vi "main_BOC.vi"() -> ()   [LabVIEW 2017]
doc: "Use this template to build a user interface event handler design pattern. Use this pattern for dialog boxes and other user interfaces. You also can create and execute user-defined events that the VI can handle the same way as user interface events."
uses:
  ui.ctl
  classes/dc_power_supply/DC_power_supply.lvclass
  classes/report/Report.lvclass
  ui_buttons.ctl
  types/boc_type.ctl
  types/tolerance_list.ctl
  types/tolerance.ctl
  subVI/motech_power_supply/types/motech_set_value_cluster.ctl
  subVI/motech_power_supply/types/channels_enum.ctl
  Unicorn Labview Library/Control/unicorn_Param.ctl
  Unicorn Labview Library/Control/unicorn_conn.ctl
  Unicorn Labview Library/Control/unicorn_JSON.ctl
  Unicorn Labview Library/Control/unicorn_ParamInt.ctl
  Unicorn Labview Library/Control/unicorn_Telemetry.ctl
  Unicorn Labview Library/Control/unicorn_Table.ctl
  Unicorn Labview Library/Control/unicorn_ParamFloat.ctl
  states_enum.ctl
  classes/dc_power_supply/motech-pps-1200/Motech-pps-1200.lvclass
  types/calibr_table_rows.ctl
  <instrlib>/PICOTEST M352XA/Public/Controls/Function.ctl
  classes/report/Report.lvclass/Report.ctl
  Unicorn Labview Library/Unicorn Library.lvlib
  <instrlib>/Siglent SDG X Series/Siglent SDG X Series.lvlib
panel:
  in  "export_report":bool
  in  "report":path
  in  "template":path
  in  "dc_power_supply":refnum<visa-resource-name>="MOTECH_DC_power_supply" caption="Источник DC"
  in  "channel_timeout_sec":dbl=15.0
  in  "voltmetr":refnum<visa-resource-name>="USB0::0x164E::0x0DAD::TW00054344::INSTR" caption="Вольтметр"
  in  "generator":refnum<visa-resource-name>="generator" caption="Генератор"
  in  "UI":T1
  out "error out":errorcluster
  out "Con":bool
  in  "Tab Control":T4(tab)
  out "Waveform Graph - Dark 2":waveform(sgl)[](graph)
  out "Slide 2":u8(slide) scale=0.0..100.0
  out "Slide":u8(slide) scale=0.0..100.0
  out "Waveform Graph - Dark":waveform(sgl)[](graph)
  in  "VersionControl":bool
  out "output array":sgl[][](array[numeric])
  in  "Array":dbl[][](array[numeric]) format="%_4p"
  in  "calibration":bool
  in  "check_calibr":bool
  in  "tolerance_list":T5=[{"MIN"="-(0.01+0.26*x)", "MAX"="(0.01+0.06*x)"}, {"MIN"="-(0.01+0.09*x)", "MAX"="(0.01+0.06*x)"}, {"MIN"="-(0.01+0.05*x)", "MAX"="(0.01+0.01*x)"}, {"MIN"="-(0.01+0.01*x)", "MAX"="(0.01+0.01*x)"}, {"MIN"="-(0.01+0.01*x)", "MAX"="(0.01+0.01*x)"}, {"MIN"="-(0.01+0.01*x)", "MAX"="(0.01+0.01*x)"}, {"MIN"="-(0.01+0.01*x)", "MAX"="(0.01+0.01*x)"}, {"MIN"="-(0.01+0.11*x)", "MAX"="(0.01+0.01*x)"}]
  in  "freq_values":dbl[](array[numeric])=[0.5, 2.0, 10.0, 20.0, 160.0, 2500.0, 4600.0, 4800.0] caption="Диапозон частот" min=0.0
  in  "freq_character":bool caption="Частотная характеристика"
  out "result_table_freq":dbl[][](array[numeric]) format="%#_4p"
  out "Array 2":bool[][](array[boolean])
  in  "tolerance_list 2":T5=[{"MIN"="-(0.01+0.01*x)", "MAX"="(0.01+0.01*x)"}, {"MIN"="-(0.01+0.01*x)", "MAX"="(0.01+0.01*x)"}, {"MIN"="-(0.01+0.01*x)", "MAX"="(0.01+0.01*x)"}, {"MIN"="-(0.01+0.01*x)", "MAX"="(0.01+0.01*x)"}, {"MIN"="-(0.01+0.01*x)", "MAX"="(0.01+0.01*x)"}, {"MIN"="-(0.01+0.01*x)", "MAX"="(0.01+0.01*x)"}, {"MIN"="-(0.01+0.01*x)", "MAX"="(0.01+0.01*x)"}, {"MIN"="-(0.01+0.01*x)", "MAX"="(0.01+0.01*x)"}]
  in  "volt_values":dbl[](array[numeric])=[5.0, 10.0, 14.0] caption="Диапозон напряжений" min=0.0
  out "check_volt_result":bool[][](array[boolean])
  in  "volt_meas":bool
  out "F-format string 2":string[][](array[string])
  in  "meas_low_voltage_ac_char":bool
  in  "tolerance_list 4":T5=[{"MIN"="-(0.01+0.01*x)", "MAX"="(0.01+0.01*x)"}, {"MIN"="-(0.01+0.01*x)", "MAX"="(0.01+0.01*x)"}, {"MIN"="-(0.01+0.01*x)", "MAX"="(0.01+0.01*x)"}, {"MIN"="-(0.01+0.01*x)", "MAX"="(0.01+0.01*x)"}, {"MIN"="-(0.01+0.01*x)", "MAX"="(0.01+0.01*x)"}, {"MIN"="-(0.01+0.01*x)", "MAX"="(0.01+0.01*x)"}, {"MIN"="-(0.01+0.01*x)", "MAX"="(0.01+0.01*x)"}, {"MIN"="-(0.01+0.01*x)", "MAX"="(0.01+0.01*x)"}]
  in  "volt_values 2":dbl[](array[numeric])=[0.005, 0.1, 1.0] caption="Диапозон напряжений" min=0.0
  out "check_volt_result 2":bool[][](array[boolean])
  out "F-format string":string[][](array[string])
  out "Table Control":string[][](table)
  in  "voltage":dbl[](array[numeric])=[-20.0, -15.0, -10.0, -5.0, -1.0, -0.1, 0.1, 1.0, 5.0, 10.0, 15.0, 20.0]
  in  "dc_voltage_measure":bool caption="connection"
  in  "tolerance_list 3":T5=[{"MIN"="-(0.01+0.01*x)", "MAX"="(0.01+0.01*x)"}, {"MIN"="-(0.01+0.01*x)", "MAX"="(0.01+0.01*x)"}, {"MIN"="-(0.01+0.01*x)", "MAX"="(0.01+0.01*x)"}, {"MIN"="-(0.01+0.01*x)", "MAX"="(0.01+0.01*x)"}, {"MIN"="-(0.01+0.01*x)", "MAX"="(0.01+0.01*x)"}, {"MIN"="-(0.01+0.01*x)", "MAX"="(0.01+0.01*x)"}, {"MIN"="-(0.01+0.01*x)", "MAX"="(0.01+0.01*x)"}, {"MIN"="-(0.01+0.01*x)", "MAX"="(0.01+0.01*x)"}]
  out "Array 3":bool[][](array[boolean])
  in  "set_V":bool
  in  "motech_set_value":T7={"voltage"=0.0, "current"=0.0, "channel"=enum."1"}
  in  "I_control_values":dbl[](array[numeric])=[4.0, 8.0, 12.0, 16.0, 20.0]
  out "first_meas":dbl[](array[numeric])
  out "result_calibration_table":sgl[][](array[numeric])
  out "second_meas":dbl[](array[numeric])
  in  "tolerance_list_I_correction":T5=[{"MIN"="-(0.1+0.01*x*1000)/1000", "MAX"="(0.1+0.01*x*1000)/1000"}, {"MIN"="-(0.1+0.01*x*1000)/1000", "MAX"="(0.1+0.01*x*1000)/1000"}, {"MIN"="-(0.1+0.01*x*1000)/1000", "MAX"="(0.1+0.01*x*1000)/1000"}, {"MIN"="-(0.1+0.01*x*1000)/1000", "MAX"="(0.1+0.01*x*1000)/1000"}, {"MIN"="-(0.1+0.01*x*1000)/1000", "MAX"="(0.1+0.01*x*1000)/1000"}, {"MIN"="-(0.01+0.01*x)", "MAX"="(0.01+0.01*x)"}, {"MIN"="-(0.01+0.01*x)", "MAX"="(0.01+0.01*x)"}, {"MIN"="-(0.01+0.11*x)", "MAX"="(0.01+0.01*x)"}]
  out "check_result":bool[][](array[boolean])
  out "result_table":dbl[][](array[numeric])
  in  "curent_calibr":bool
  in  "avarage_Ac_input":bool
  in  "voltage 2":dbl[](array[numeric])=[20.0, 15.0, 10.0, 5.0, 1.0, 0.1, 0.0, 0.0, 0.0, 0.0, 0.0, 0.0]
  out "Table Control 2":string[][](table)
  in  "check_dc_icp":bool
  out "output array 2":dbl[][](array[numeric]) format="%#_6f"
  out "boc_values":sgl[][](array[numeric]) format="%#_6f"
  in  "connection":bool
  in  "stop":bool
  # "Данные при калибровке"
  # "Проверка калибровки"
  # "dc_before"
  # "rms_before"
  # "measured"
  # "dc_result"
  # "rms_result"
  # "dc_after"
  # "rms_after"
  # "abs_before (%)"
  # "abs_after (%)"
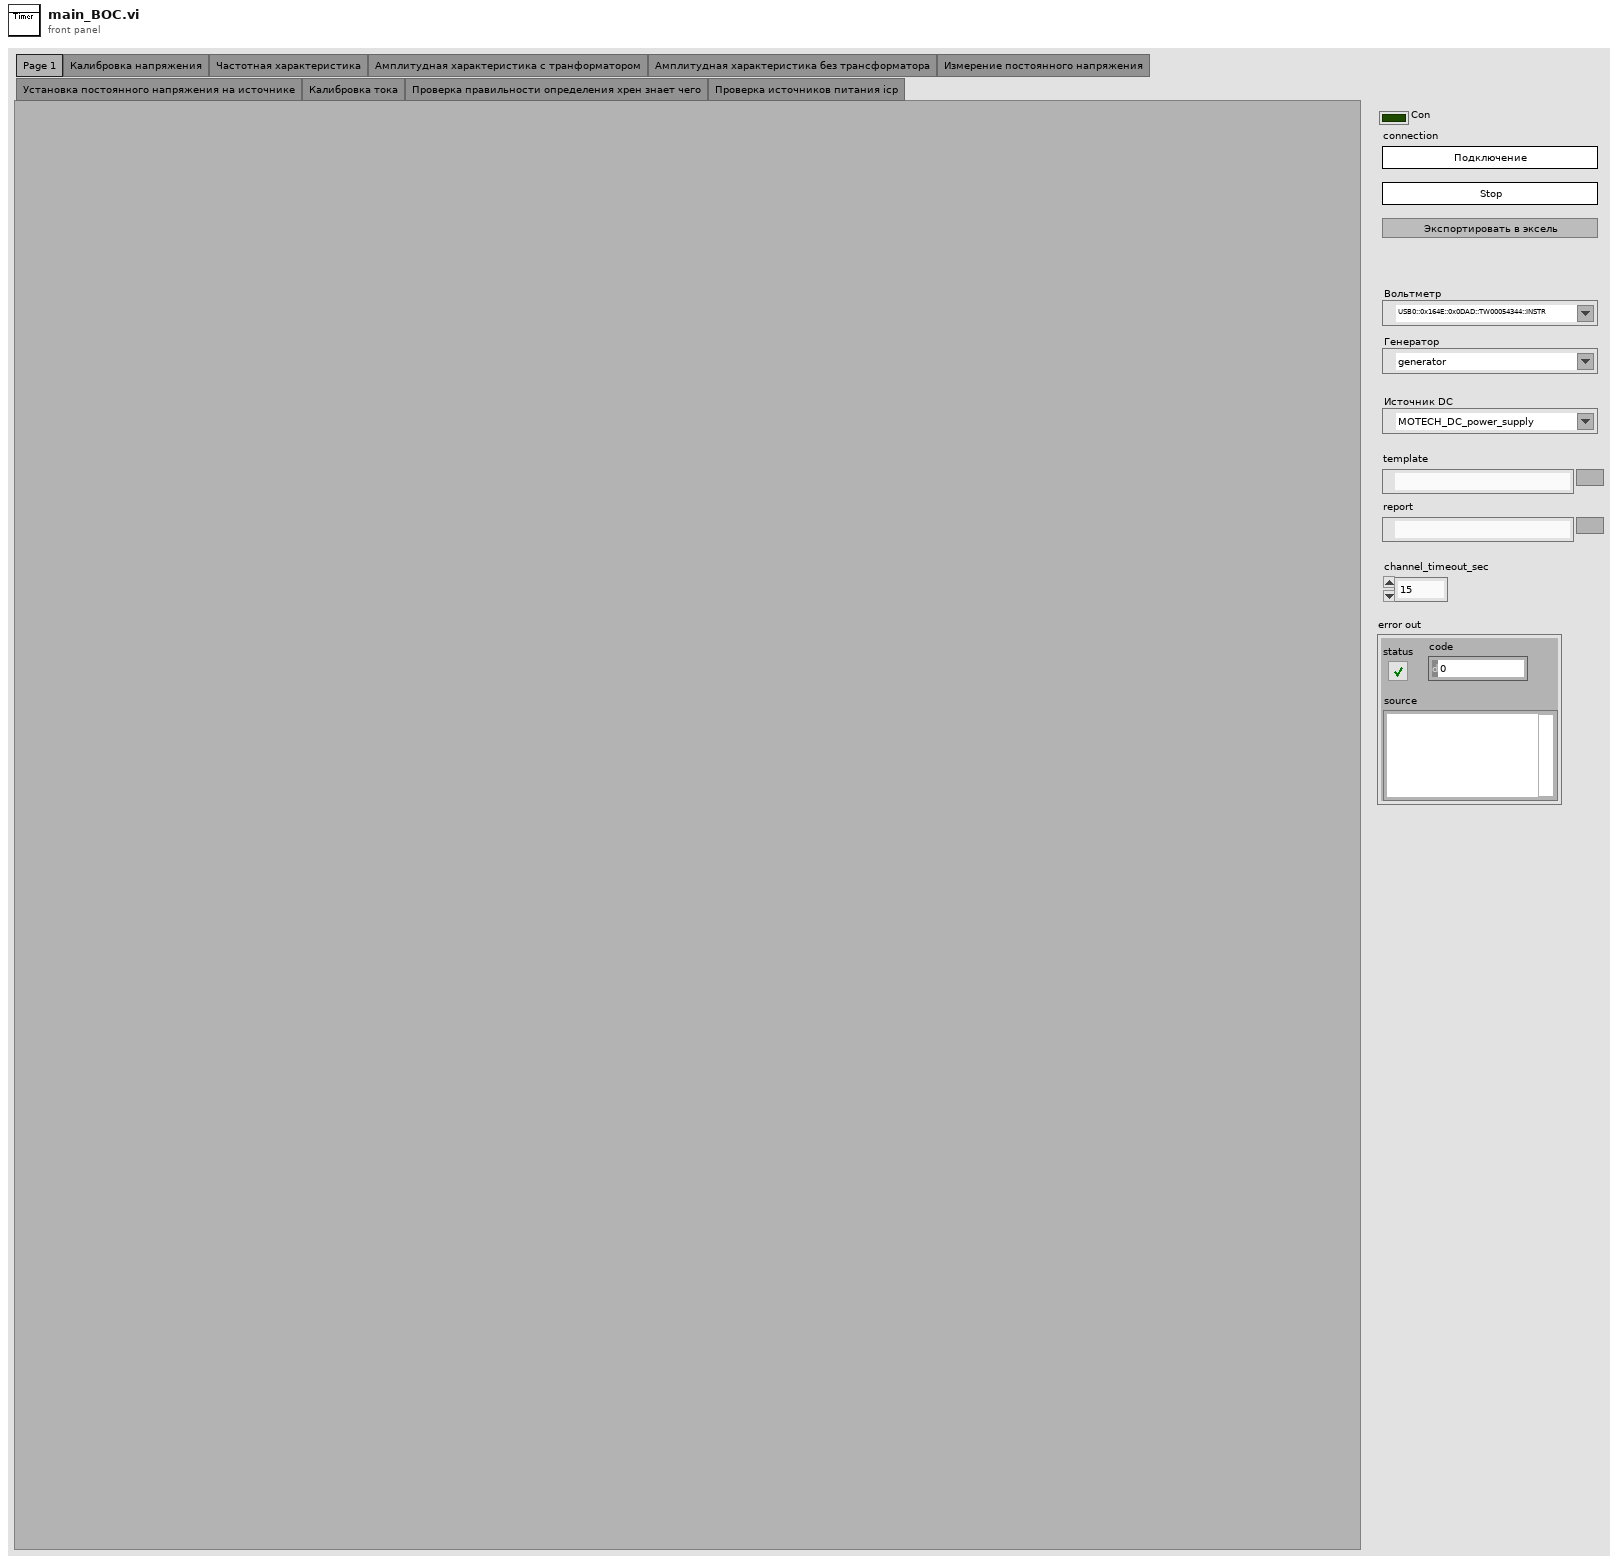
[diagram p1: front panel]
types:
  T1 = typedef "ui.ctl" = cluster{"UI_buttons":T2, "Tab Control":refnum<vi>, "connect_button":refnum<vi>, "generator":refnum<visa-resource-name>, "voltmetr":refnum<visa-resource-name>, "channel_timeout_sec":dbl, "boc_type":T3, "result_array_":refnum<vi>, "DC_power_supply.lvclass":refnum<class "DC_power_supply.lvclass">, "Report.lvclass":refnum<class "Report.lvclass">, "report_template":refnum<vi>, "report":refnum<vi>}
  T2 = typedef "ui_buttons.ctl" = refnum<vi>[]
  T3 = typedef "boc_type.ctl" = enum16{"БОЦ-6", "БОЦ-12"}
  T4 = enum32{"Page 1", "Калибровка напряжения", "Частотная характеристика", "Амплитудная характеристика с транформатором", "Амплитудная характеристика без трансформатора", "Измерение постоянного напряжения", "Установка постоянного напряжения на источнике", "Калибровка тока", "Проверка правильности определения хрен знает чего", "Проверка источников питания icp"}
  T5 = typedef "tolerance_list.ctl" = T6[]
  T6 = typedef "tolerance.ctl" = cluster{"MIN":string, "MAX":string}
  T7 = typedef "motech_set_value_cluster.ctl" = cluster{"voltage":dbl, "current":dbl, "channel":T8}
  T8 = typedef "channels_enum.ctl" = enum16{"0", "1", "2"}
  T9 = typedef "states_enum.ctl" = enum16{"init", "process", "exit"}
  T10 = typedef "Unicorn Library.lvlib/unicorn_Param.ctl" = cluster{"conParam":T11, "Param":T12}
  T11 = typedef "Unicorn Library.lvlib/unicorn_conn.ctl" = cluster{"ReadIntParam":bool, "ReadDescrParam":bool, "ReadFloatParam":bool, "debug":bool, "ReadJSON":bool, "IP_address":string, "N_attempts":i32, "type_con":enum16{"Serial", "TCP"}, "MB_address":i32, "VISA":refnum<visa-resource-name>, "connection ID":refnum<k5>, "nameDevices":string, "timeout":i32, "port":u16, "type_version":string, "baud_rate":u32, "VersionControl":bool, "TCP_conn":bool, "WindowSize":i32}
  T12 = typedef "Unicorn Library.lvlib/unicorn_JSON.ctl" = cluster{"NumParam":cluster{"NTelem":i32, "NInt":i32, "NFloat":i32, "NTable":i32}, "ParamInt":T13, "Telemetry":T14, "Table":T15, "ParamFloat":T16}
  T13 = typedef "Unicorn Library.lvlib/unicorn_ParamInt.ctl" = cluster{"ID":string, "Num":i32, "Name":string, "Type":string, "Enum":string, "Desc":string, "Unit":string, "Access":string, "FormatStr":string, "Min":i32, "Max":i32}[]
  T14 = typedef "Unicorn Library.lvlib/unicorn_Telemetry.ctl" = cluster{"ID":string, "Num":i32, "Name":string, "Desc":string, "Unit":string, "FormatStr":string, "Min":i32, "Max":i32}[]
  T15 = typedef "Unicorn Library.lvlib/unicorn_Table.ctl" = cluster{"Num":i32, "Access":string, "ColumnCount":i32, "NeedParamPrepare":bool, "Columns":cluster{"Column":i32, "Desc":string, "Name":string}[], "DataType":string, "FormatStr":string, "ID":string, "Name":string, "RowCount":i32, "Rows":cluster{"Desc":string, "ID":string, "Max":i32, "Min":i32, "Name":string, "Row":i32, "Unit":string}[], "Type":string}[]
  T16 = typedef "Unicorn Library.lvlib/unicorn_ParamFloat.ctl" = cluster{"ID":string, "Num":i32, "Name":string, "Type":string, "Enum":string, "Desc":string, "Unit":string, "Access":string, "FormatStr":string, "Min":i32, "Max":i32}[]
  T17 = typedef "calibr_table_rows.ctl" = enum16{"dc_before", "rms_before", "measured", "dc_result", "rms_result", "dc_after", "rms_after", "abs_before", "abs_after"}
  T18 = typedef "Function.ctl" = enum16{"VOLTage:DC", "VOLTage:DC:RATio", "VOLTage:AC", "CURRent:DC", "CURRent:AC", "RESistance", "FRESistance", "FREQuency", "PERiod", "FREQuency:CURRent", "PERiod:CURRent", "CAPacitance", "CONTinuity", "DIODe", "TCOuple", "TEMPerature"}
  T19 = cluster{"positive_channel":T8, "negative_channel":T8}
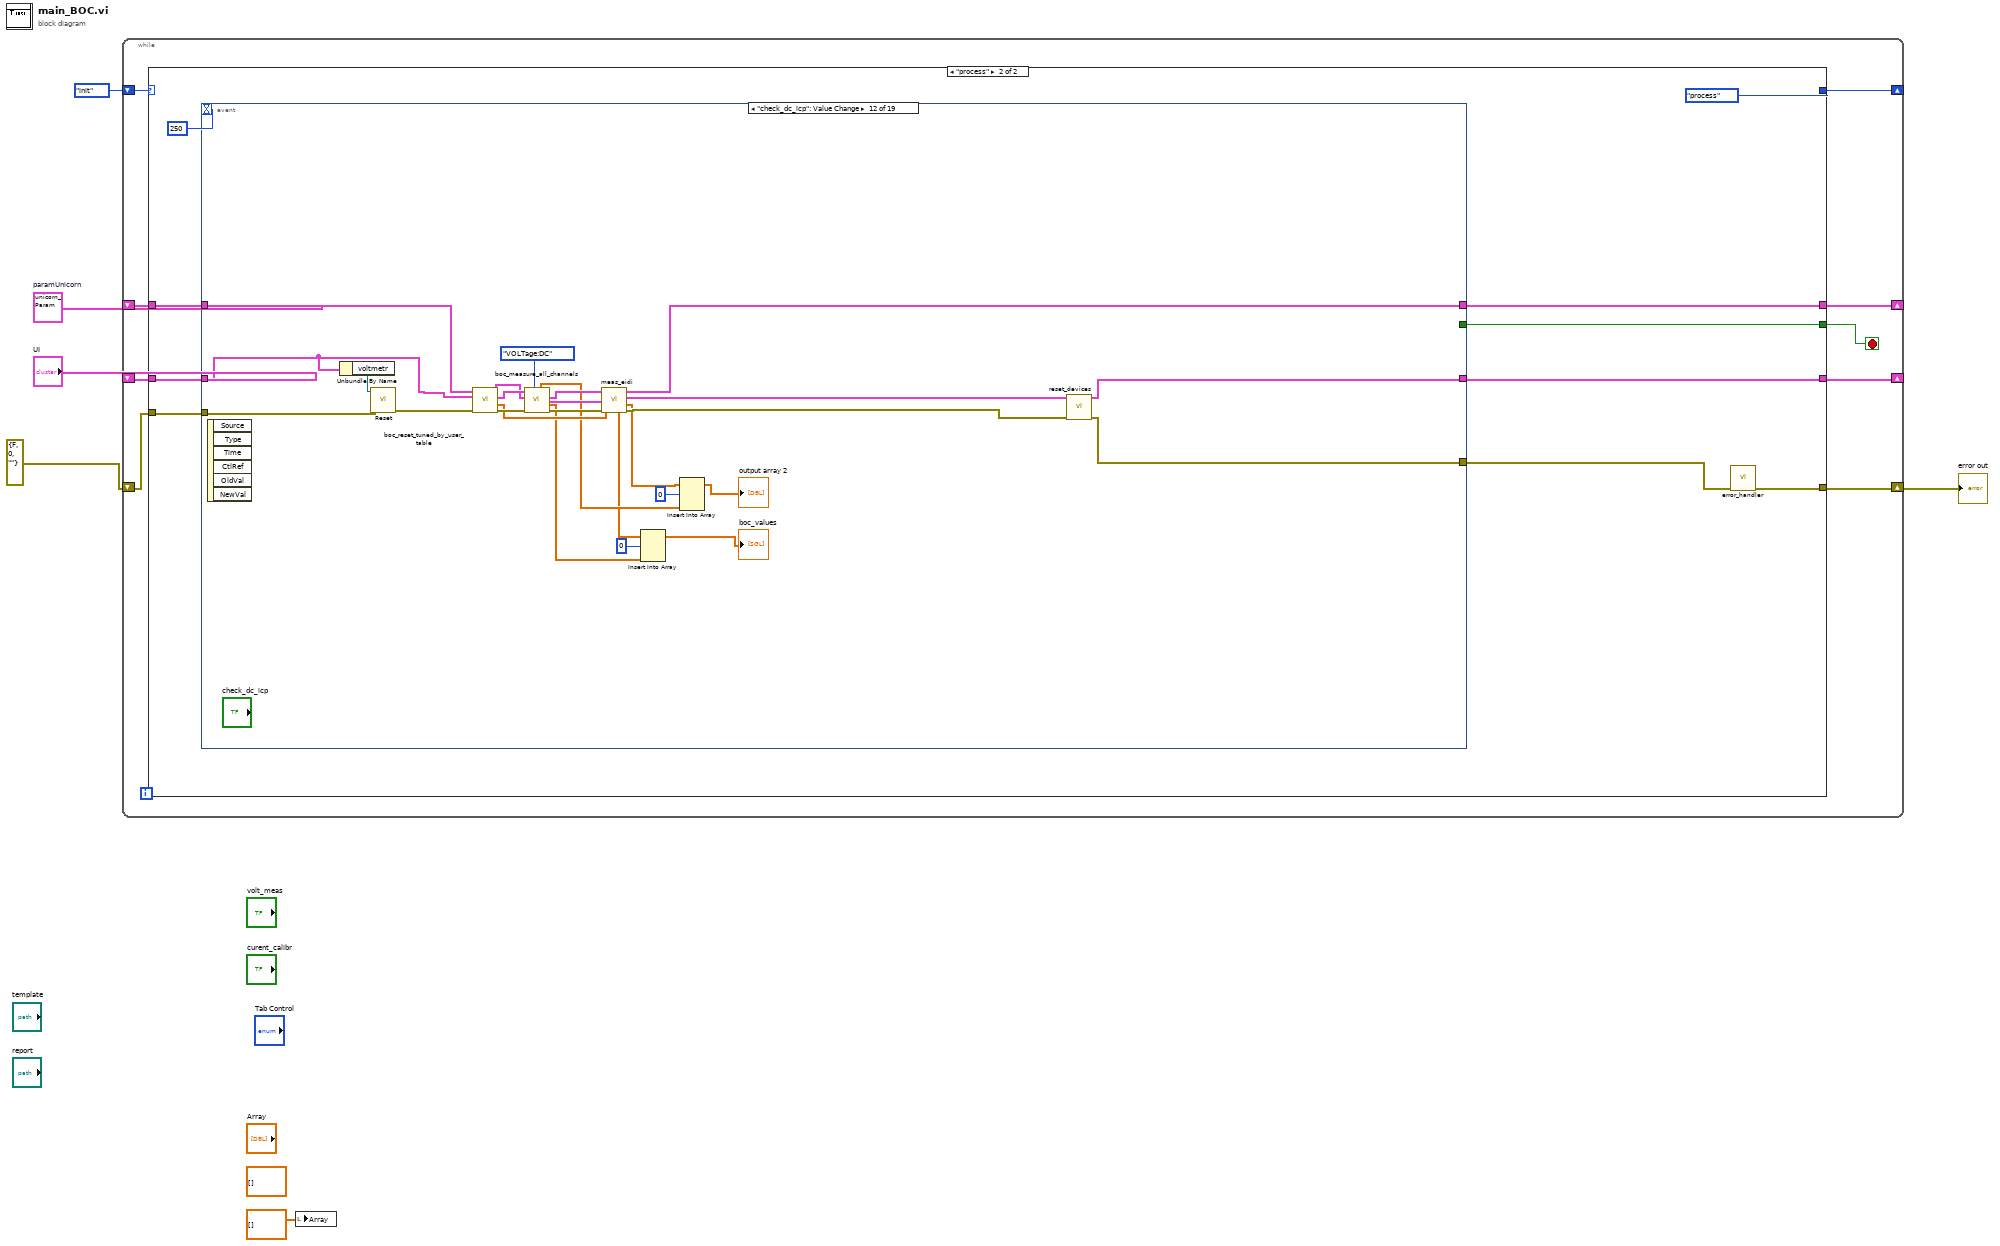
[diagram p0: block diagram]
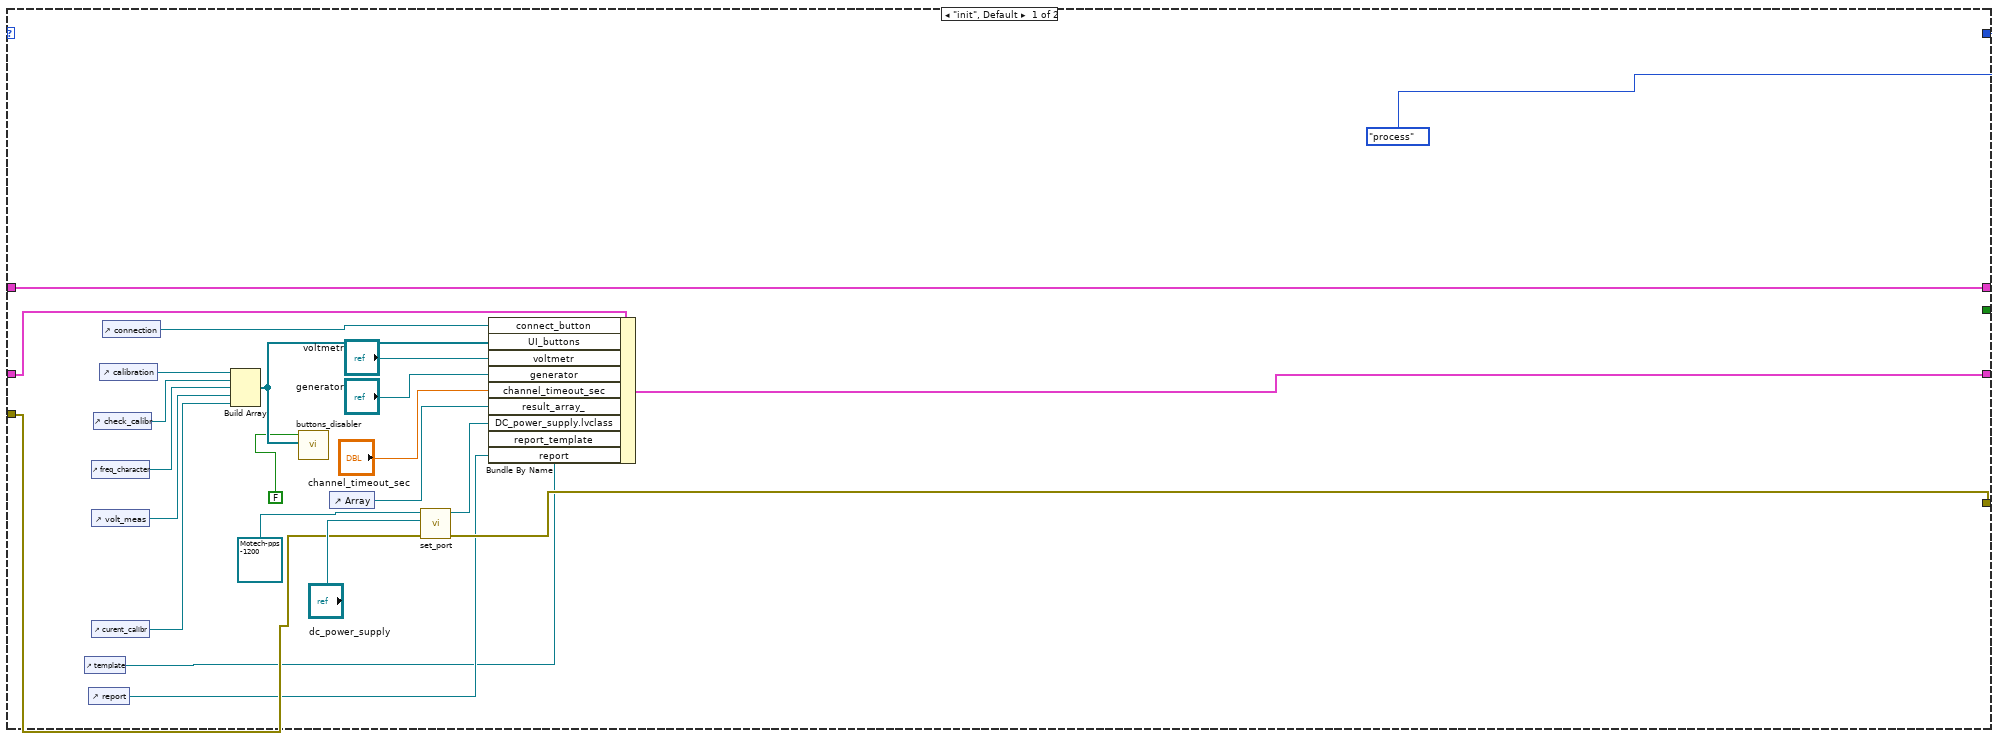
[diagram p2: hidden frame]
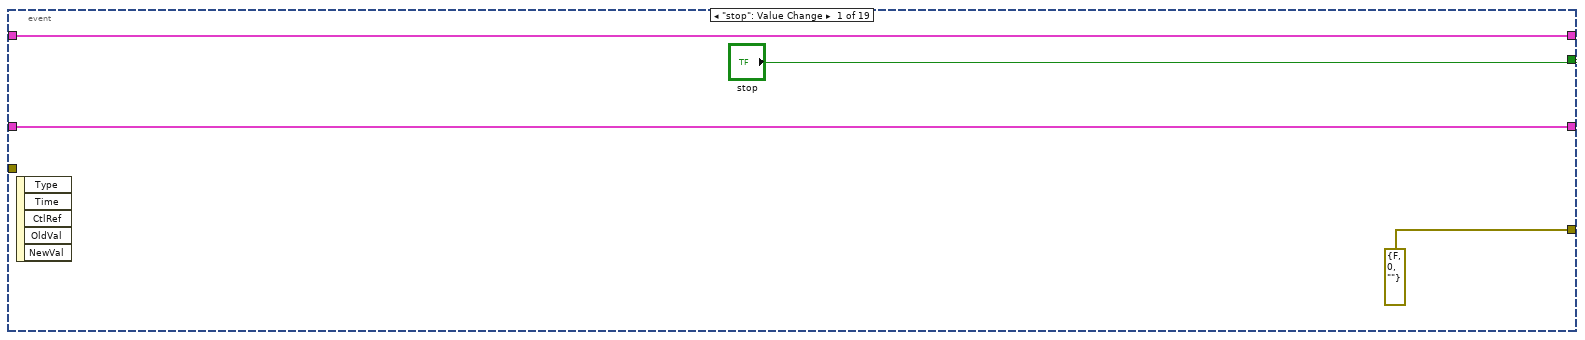
[diagram p3: hidden frame]
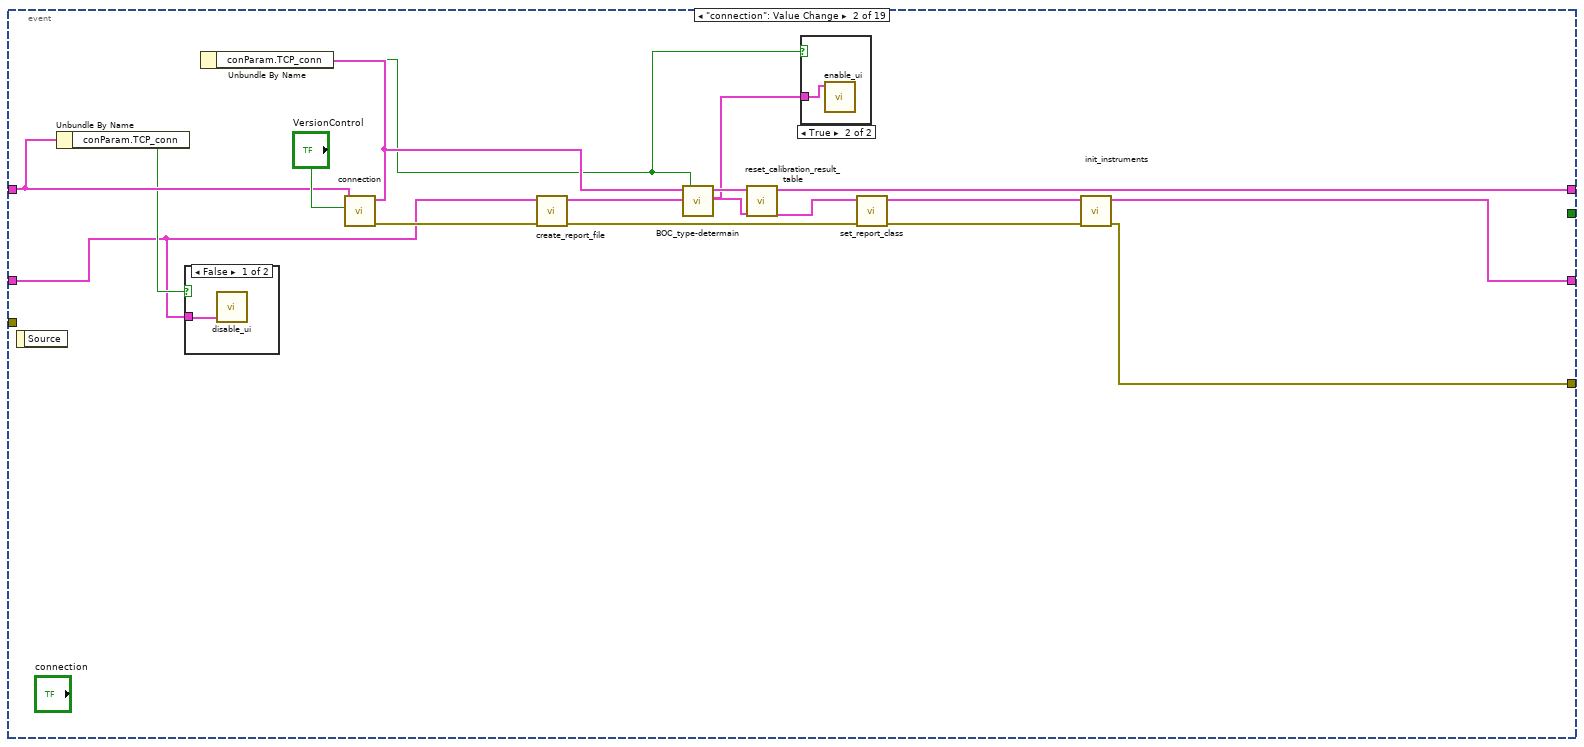
[diagram p4: hidden frame]
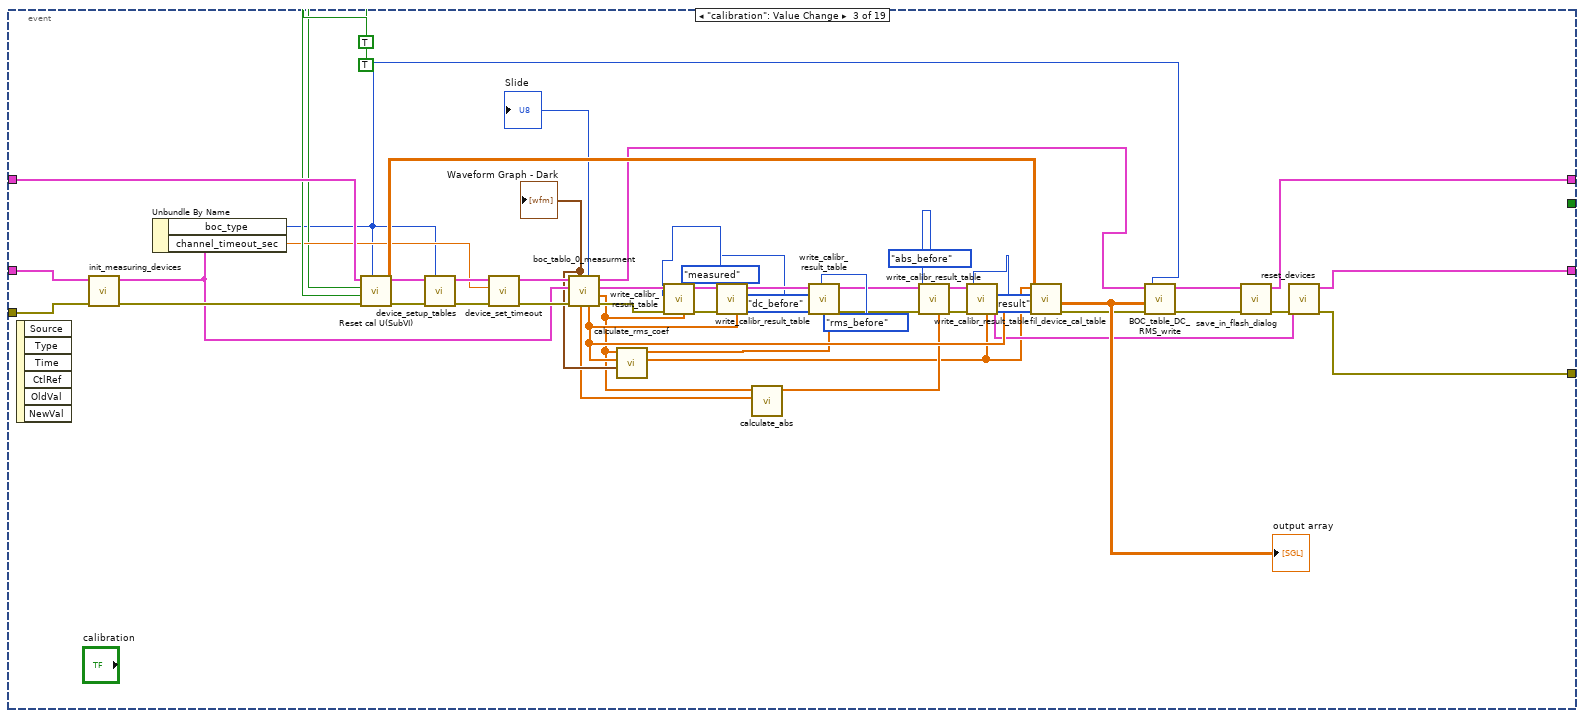
[diagram p7: hidden frame]
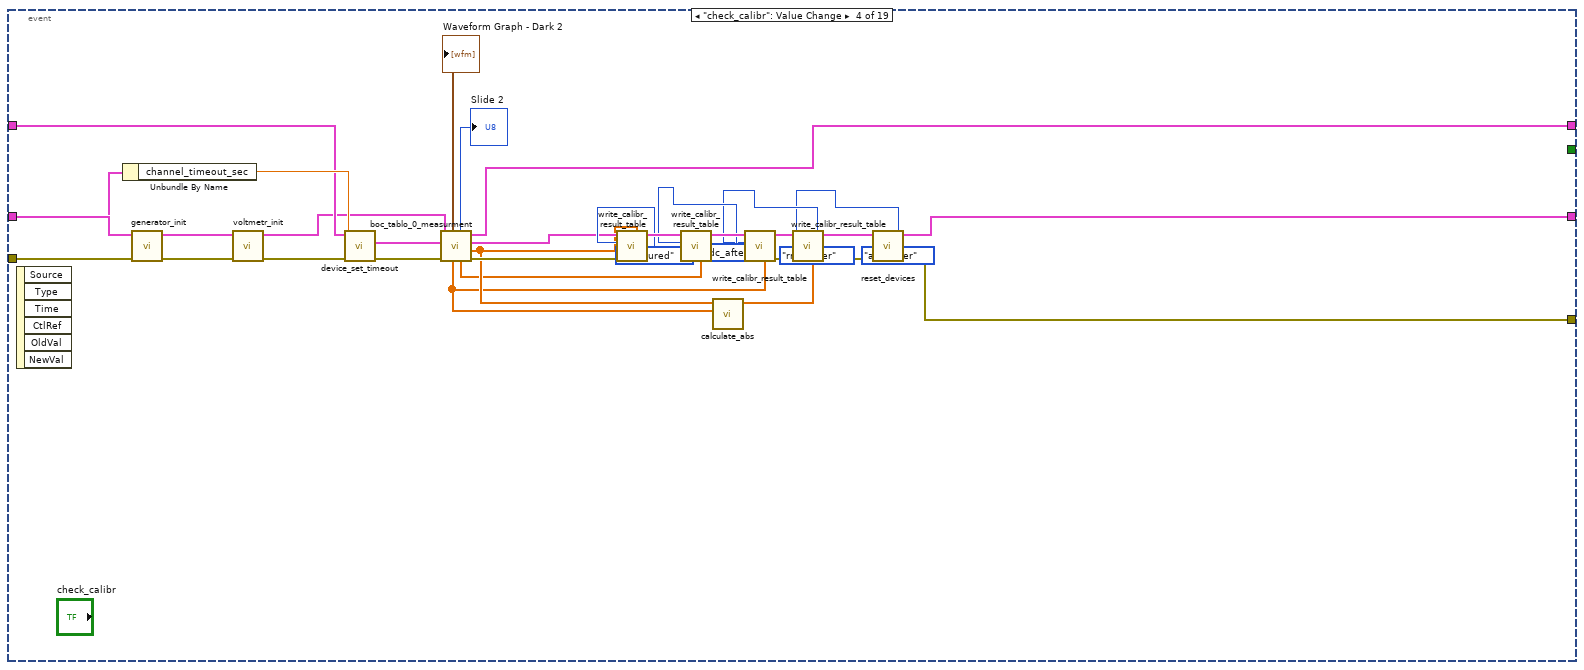
[diagram p8: hidden frame]
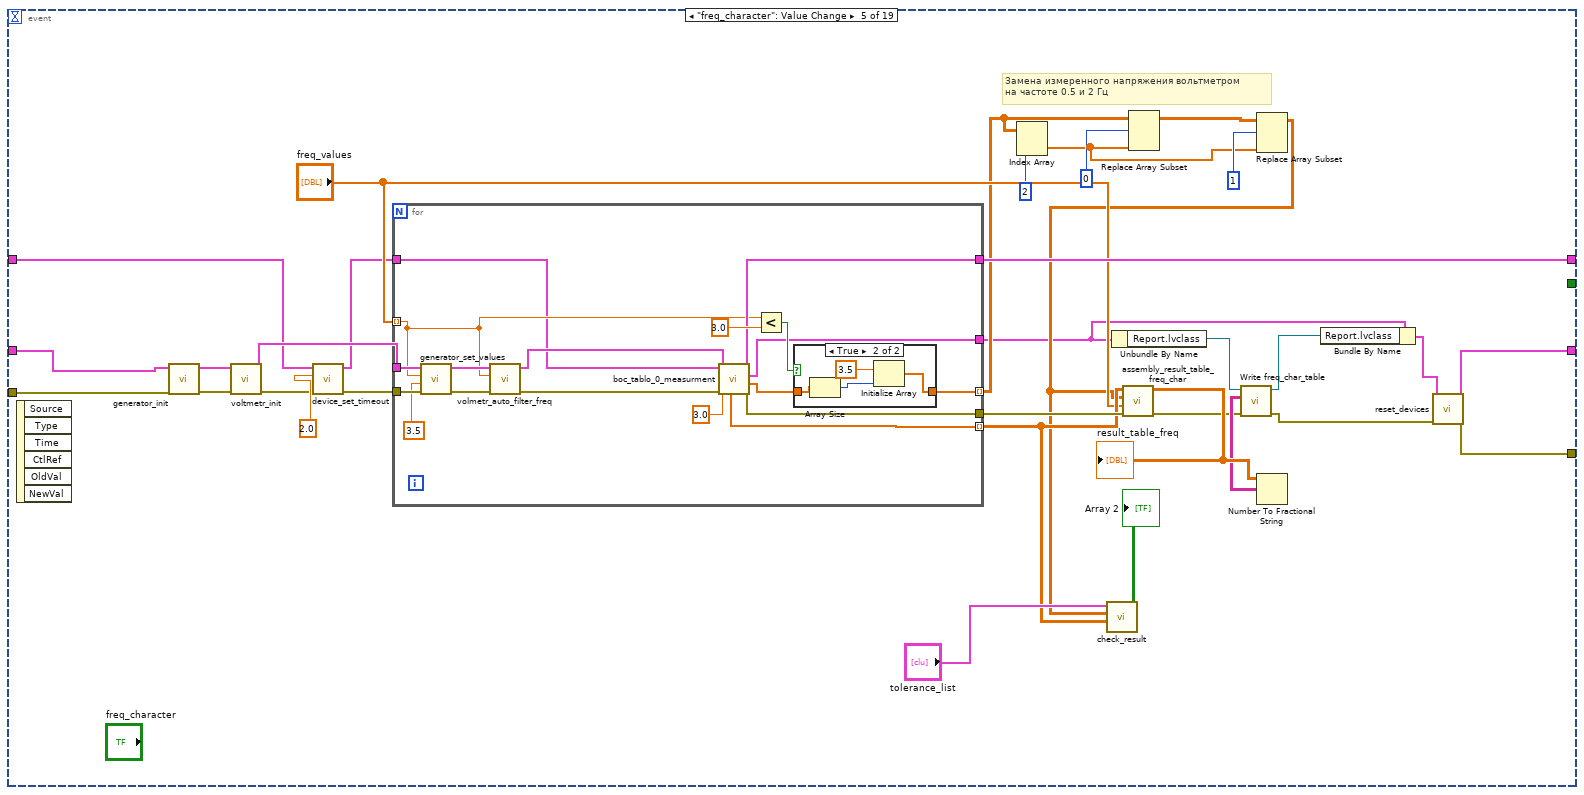
[diagram p9: hidden frame]
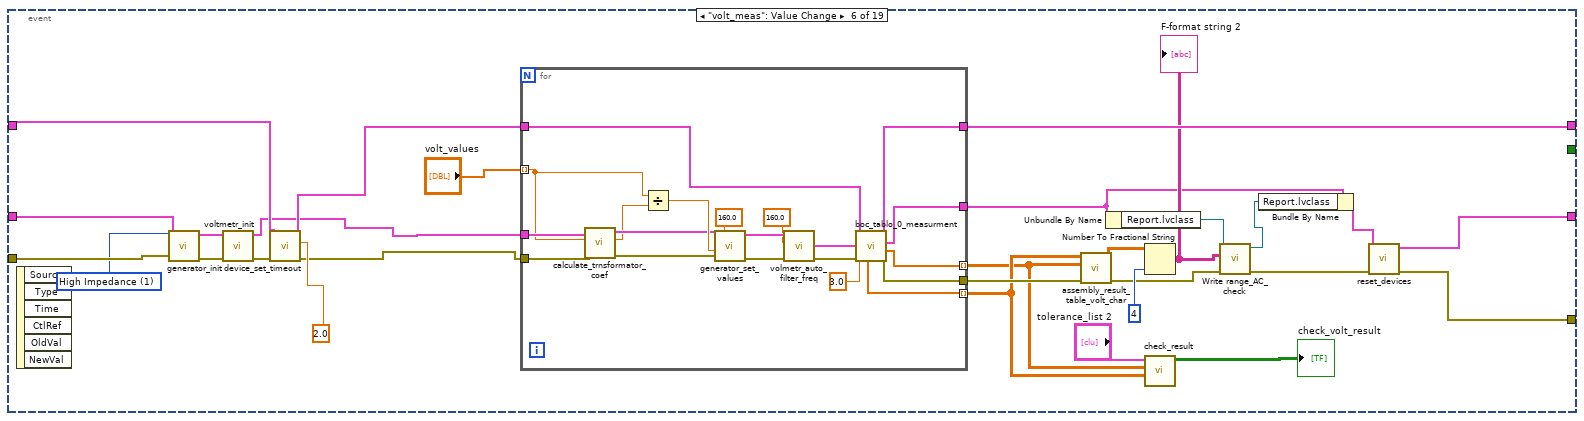
[diagram p11: hidden frame]
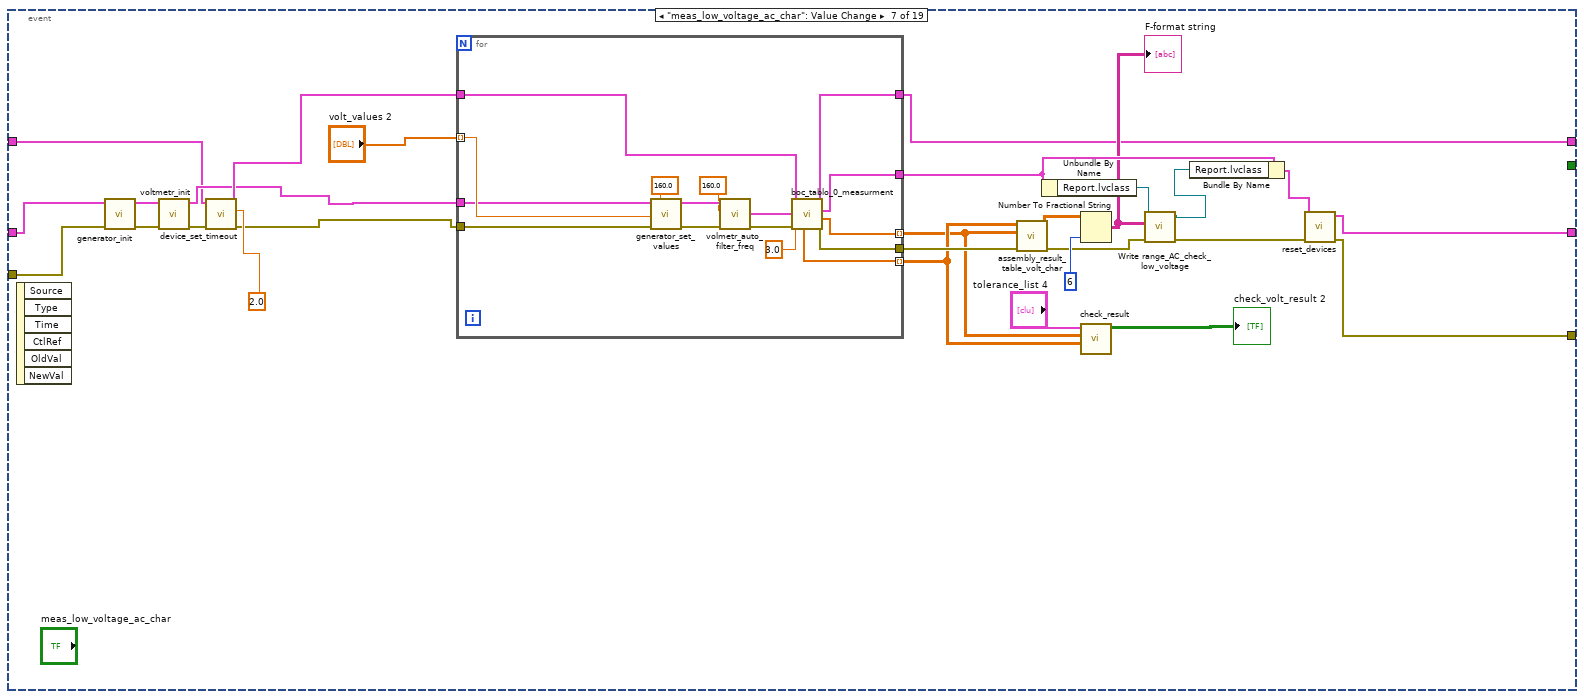
[diagram p12: hidden frame]
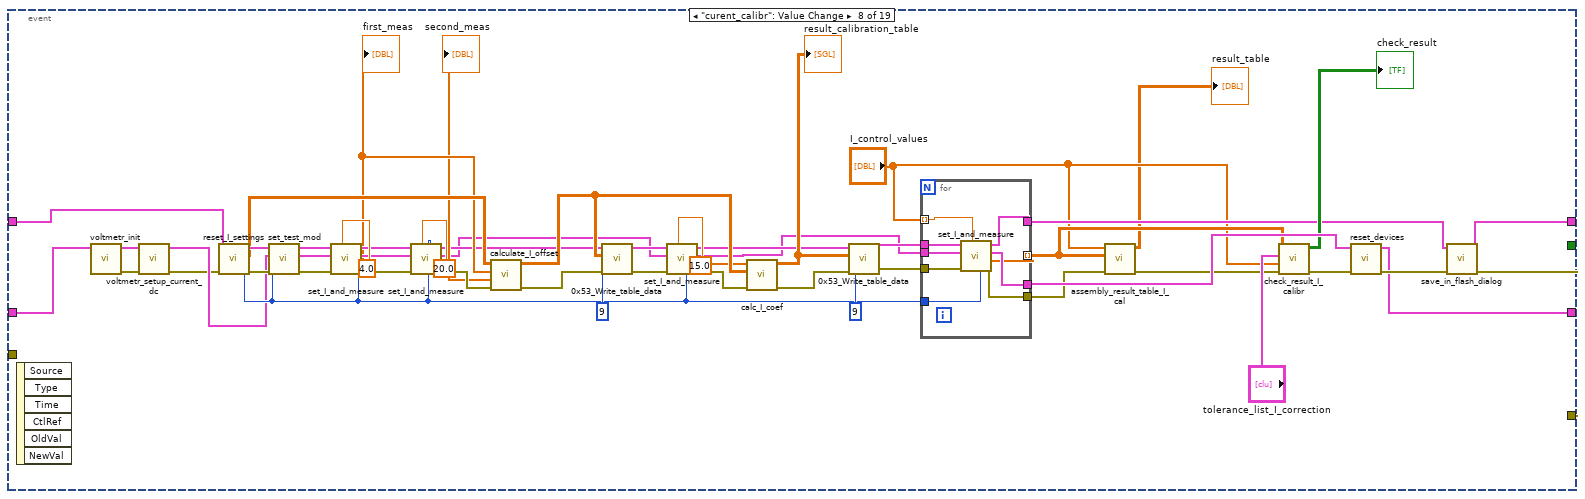
[diagram p13: hidden frame]
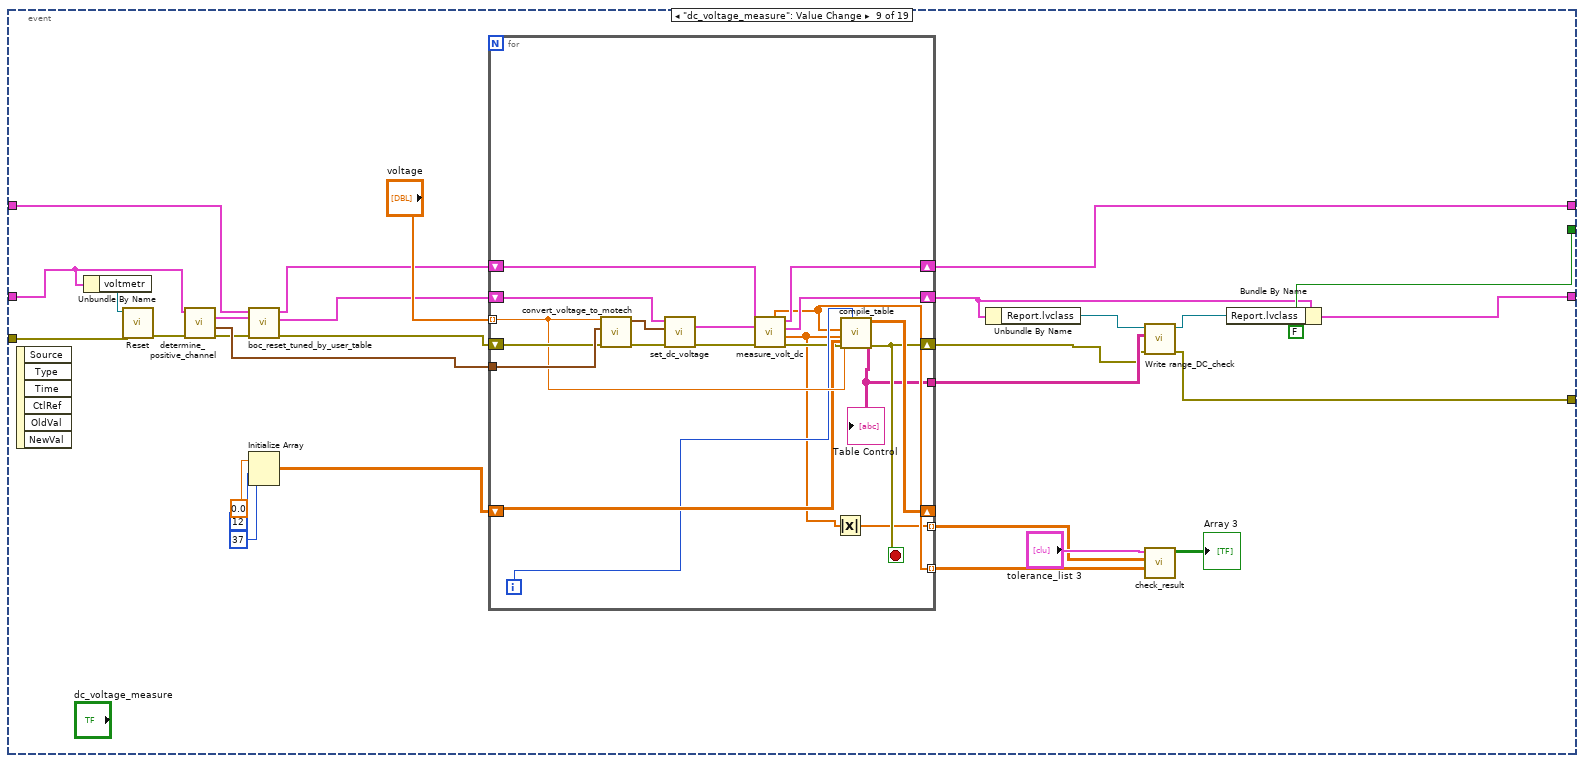
[diagram p14: hidden frame]
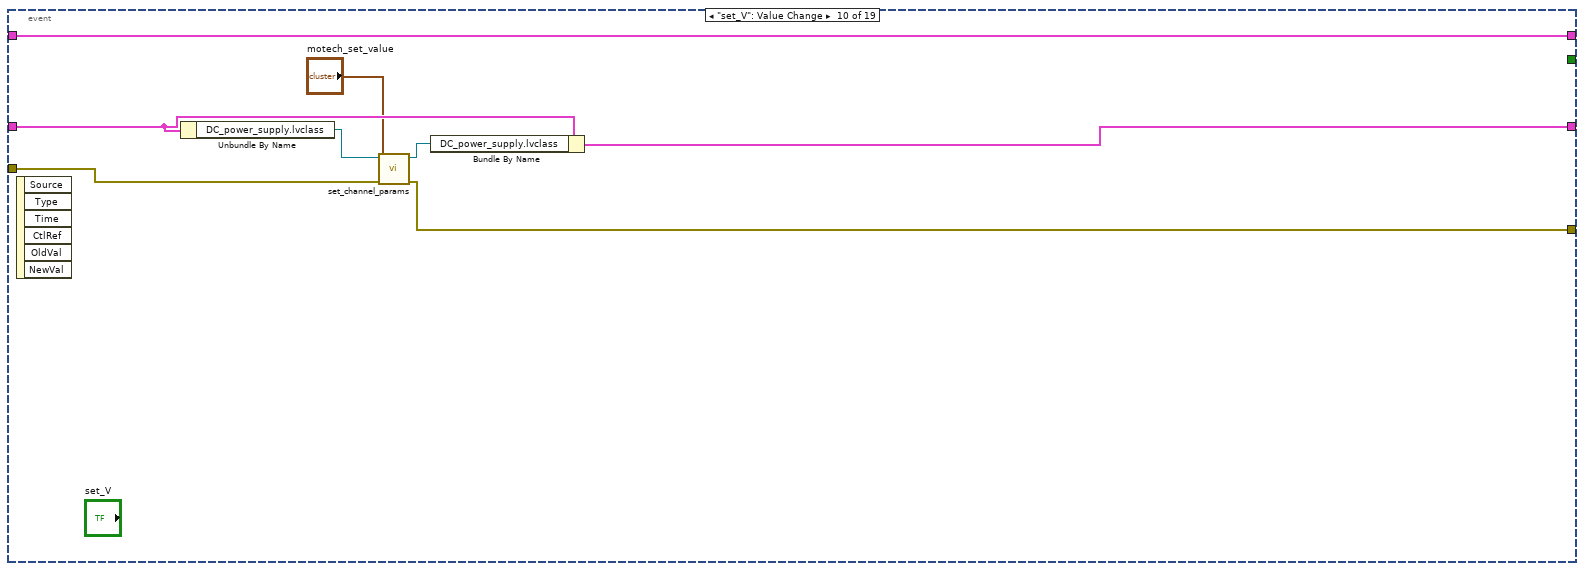
[diagram p15: hidden frame]
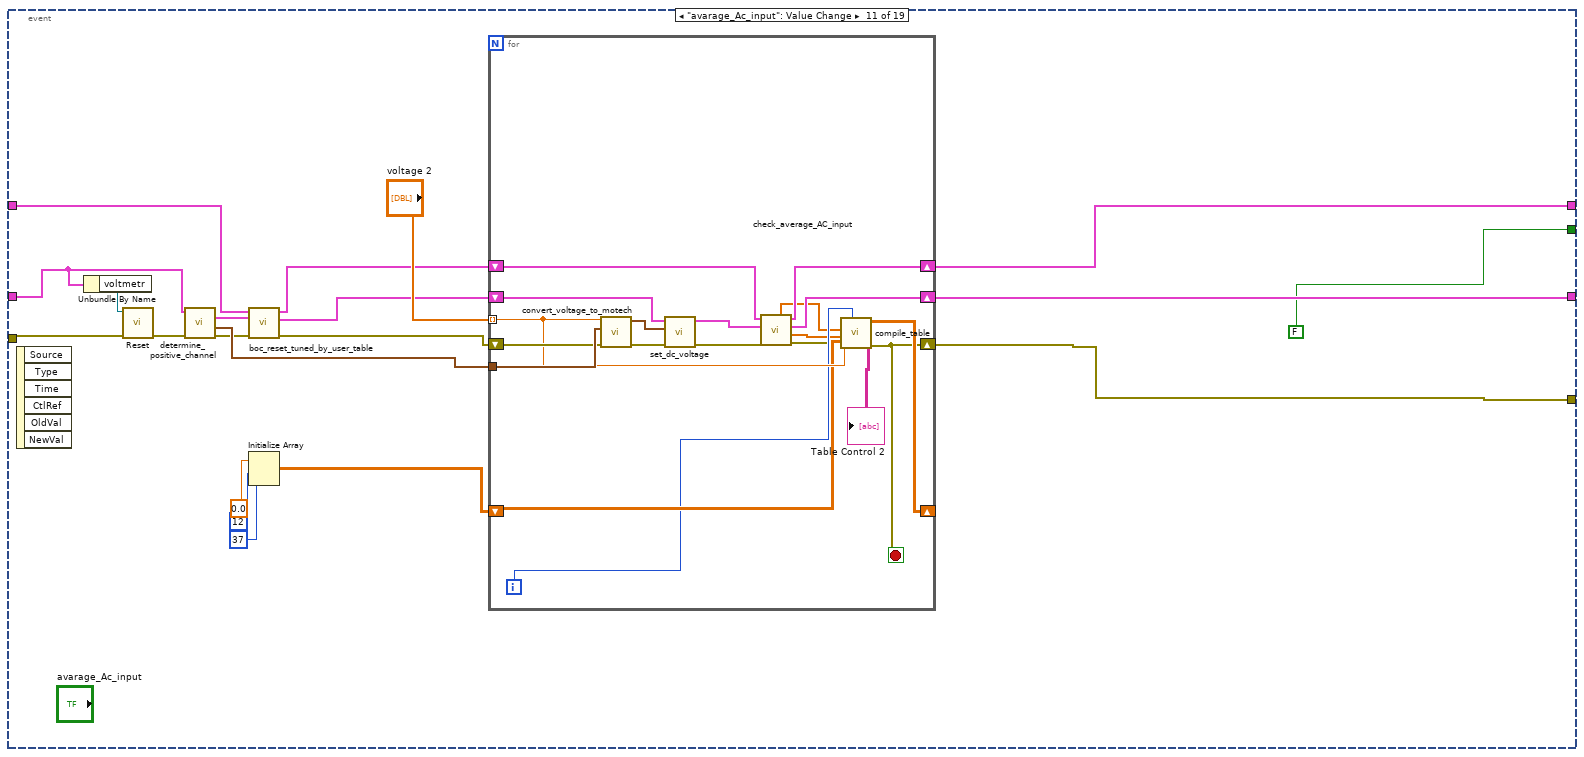
[diagram p16: hidden frame]
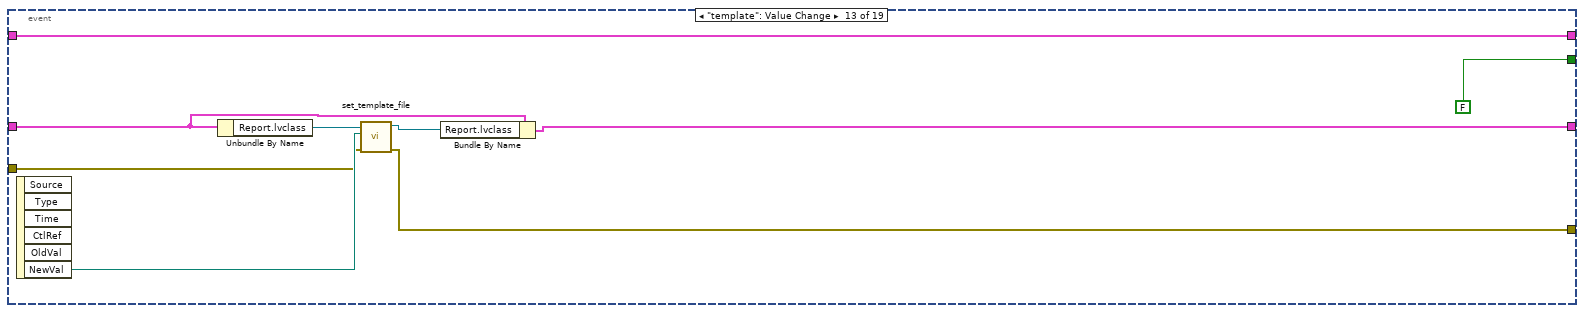
[diagram p17: hidden frame]
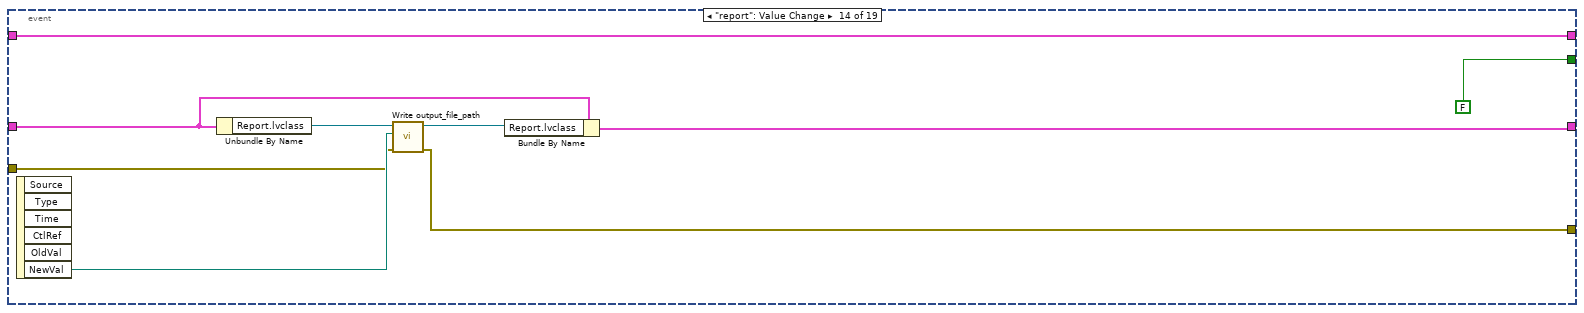
[diagram p18: hidden frame]
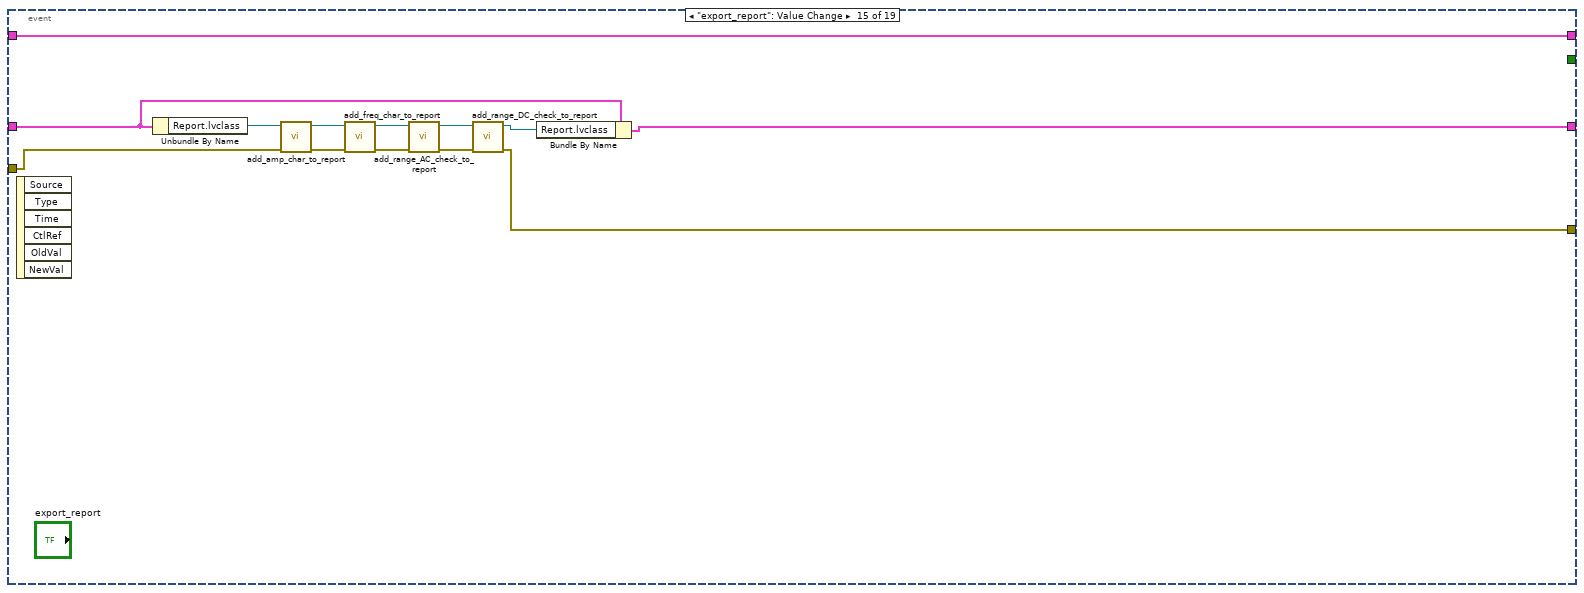
[diagram p19: hidden frame]
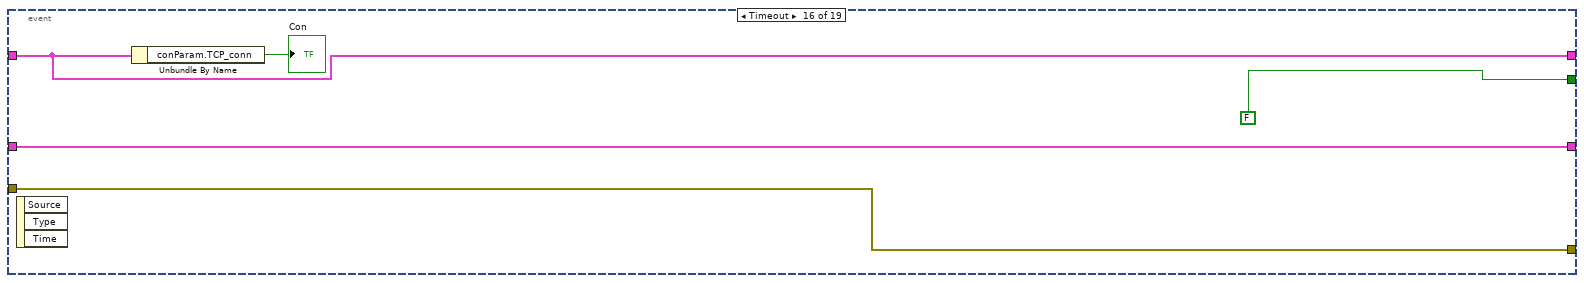
[diagram p20: hidden frame]
diagram:
  (unwired) dbl[][] [] ("Array")
  w5 = T10 {"conParam"={"ReadIntParam"=TRUE, "ReadDescrParam"=FALSE, "ReadFloatParam"=TRUE, "debug"=FALSE, "ReadJSON"=TRUE, "IP_address"="192.168.1.216", "N_attempts"=3, "type_con"=enum."TCP", "MB_address"=1, "VISA"="COM1", "connection ID"=refnum, "nameDevices"="", "timeout"=1000, "port"=2000, "type_version"="0F0C0001", "baud_rate"=115200, "VersionControl"=TRUE, "TCP_conn"=FALSE, "WindowSize"=700}, "Param"={"NumParam"={"NTelem"=201, "NInt"=16, "NFloat"=10, "NTable"=2}, "ParamInt"=[{"ID"="Режим работы", "Num"=0, "Name"="", "Type"="", "Enum"="", "Desc"="", "Unit"="", "Access"="", "FormatStr"="", "Min"=0, "Max"=0}, {"ID"="", "Num"=0, "Name"="", "Type"="", "Enum"="", "Desc"="", "Unit"="", "Access"="", "FormatStr"="", "Min"=0, "Max"=0}, {"ID"="", "Num"=0, "Name"="", "Type"="", "Enum"="", "Desc"="", "Unit"="", "Access"="", "FormatStr"="", "Min"=0, "Max"=0}, {"ID"="", "Num"=0, "Name"="", "Type"="", "Enum"="", "Desc"="", "Unit"="", "Access"="", "FormatStr"="", "Min"=0, "Max"=0}, {"ID"="", "Num"=0, "Name"="", "Type"="", "Enum"="", "Desc"="", "Unit"="", "Access"="", "FormatStr"="", "Min"=0, "Max"=0}, {"ID"="", "Num"=0, "Name"="", "Type"="", "Enum"="", "Desc"="", "Unit"="", "Access"="", "FormatStr"="", "Min"=0, "Max"=0}, {"ID"="ModeWork", "Num"=0, "Name"="", "Type"="", "Enum"="", "Desc"="", "Unit"="", "Access"="", "FormatStr"="", "Min"=0, "Max"=0}], "Telemetry"=[], "Table"=[], "ParamFloat"=[]}}  # paramUnicorn
  n1 = while {
    shift-right: [w10] -> _
    shift-left: "UI" -> [w14]
    shift-right: [w9] -> _
    shift-left: w5 -> [w12]
    shift-right: [w11] -> _
    shift-left: states_enum."init" -> [w13]
    shift-right: [w8] -> w3
    shift-left: errorcluster {"status"=FALSE, "code"=0, "source"=""} ("error in (no error)") -> [w7]
    stop <- w15 stop-if-true
    n2 = case shown="\"process\"" w13 {
      tunnel: [_ w48] -> w15
      tunnel: w14 -> [w25 w46]
      tunnel: [w30 w43] -> w9
      tunnel: w12 -> [w30 w47]
      tunnel: [states_enum."process" states_enum."process"] -> w11
      tunnel: w7 -> [w18 w44]
      tunnel: [w24 w41] -> w10
      tunnel: [w21 w40] -> w8
      frame "init", Default {
        n3 = control-ref of="template"() -> (w16:refnum<vi>)
        n4 = control-ref of="report"() -> (w17:refnum<vi>)
        n5 = control-ref of="freq_character"() -> (w35:refnum<vi>)
        n6 = control-ref of="volt_meas"() -> (w34:refnum<vi>)
        n7 = control-ref of="curent_calibr"() -> (w33:refnum<vi>)
        n8 = control-ref of="check_calibr"() -> (w36:refnum<vi>)
        n9 = control-ref of="calibration"() -> (w37:refnum<vi>)
        n10 = control-ref of="connection"() -> (w38:refnum<vi>)
        n11 = Build Array(w37, w36, w35, w34, w33) -> (w32:refnum<vi>[])
        n12 = call "buttons_disabler.vi"("Array"=w32, "s"=FALSE) -> ()  [unwired: 10 in]
        n13 = control-ref of="Array"() -> (w23:refnum<vi>)
        n14 = call-dynamic "set_port.vi"("error in (no error)"=w18, "VISA resource name"="dc_power_supply", "Motech-pps-1200 in"=refnum<class "Motech-pps-1200.lvclass"> refnum ("Motech-pps-1200.lvclass")) -> ("error out"=w21:errorcluster, "Motech-pps-1200 out"=w19:refnum<class "Motech-pps-1200.lvclass">)  [unwired: 7 in]
        n15 = Bundle By Name(cluster=w25, "connect_button"=w38, "UI_buttons"=w32, "voltmetr"="voltmetr", "generator"="generator", "channel_timeout_sec"="channel_timeout_sec", "result_array_"=w23, "DC_power_supply.lvclass"=w19, "report_template"=w16, "report"=w17) -> (w24:T1)
      }
      frame "process" {
        n16 = event shown="[11] \"check_dc_icp\": Value Change" {
          selector: _ -> [_ _ _ _ _ _ _ _ _ _ _ _ _ _ _ _ _ _ _]
          dyn-events: _ -> [_ _ _ _ _ _ _ _ _ _ _ _ _ _ _ _ _ _ _]
          timeout: 250 -> [_ _ _ _ _ _ _ _ _ _ _ _ _ _ _ _ _ _ _]
          tunnel: ["stop" _ _ _ _ _ _ _ FALSE ("stop") _ FALSE ("stop") _ FALSE ("stop") FALSE ("stop") _ FALSE ("stop") _ _ _] -> w48
          tunnel: w46 -> [w50 w62 w109 w148 w185 w221 w261 w342 w386 w419 w422 w471 w492 w501 w513 w521 w527 w537 w544]
          tunnel: w47 -> [w51 w66 w118 w146 w164 w225 w260 w355 w383 w417 w428 w485 w488 w497 w505 w520 w523 w535 w538]
          tunnel: [w51 w67 w104 w145 w182 w235 w263 w316 w392 w417 w423 w476 w488 w497 w505 w520 w523 w535 w538] -> w43
          tunnel: w44 -> [_ _ w119 w149 w183 w220 w262 _ w387 w416 w427 w484 w493 w502 w511 w519 w528 w533 w541]
          tunnel: [w50 w61 w72 w144 w181 w214 w264 w305 w366 w418 w425 w473 w490 w498 w506 w521 w525 w536 w539] -> w41
          tunnel: [errorcluster {"status"=FALSE, "code"=0, "source"=""} ("error out") w60 w73 w122 w178 w234 w265 w304 w368 w415 w426 w472 w489 w499 w507 w519 w524 w531 w540] -> w39
          event "stop": Value Change {
            n17 = event-data() -> ()  [unwired: 1 in, 5 out]
          }
          event "connection": Value Change {
            n18 = event-data() -> ()  [unwired: 1 in, 1 out]
            n19 = Unbundle By Name(w66) -> ("conParam.TCP_conn"=w65:bool)
            n20 = case shown="False" w65 {
              tunnel: w62 -> [w71 _]
              frame False {
                n21 = call "disable_ui.vi"("UI"=w71) -> ()  [unwired: 11 in]
              }
              frame True {
              }
            }
            n22 = call "connection.vi"("VersionControl"="VersionControl", "paramUnicorn in"=w66) -> ("error out"=w63:errorcluster, "paramUnicorn out"=w68:T10)  [unwired: 8 in]
            n23 = Unbundle By Name(w68) -> ("conParam.TCP_conn"=w59:bool)
            n24 = call "create_report_file.vi"("error in (no error)"=w63, "UI"=w62) -> ("error out"=w57:errorcluster, "output cluster"=w54:T1)  [unwired: 8 in]
            n25 = call "BOC_type-determain.vi"("paramUnicorn_in"=w68, "UI_in"=w54, "TCP_conn"=w59) -> ("paramUnicorn_out"=w64:T10, "UI_out"=w53:T1)  [unwired: 5 in]
            n26 = call "reset_calibration_result_table.vi"("UI_in"=w53, "paramUnicorn_in"=w64) -> ("UI_out"=w58:T1, "paramUnicorn_out"=w67:T10)  [unwired: 8 in]
            n27 = case shown="True" w59 {
              tunnel: w53 -> [_ w70]
              frame False {
              }
              frame True {
                n28 = call "enable_ui.vi"("UI_out"=w70) -> ()  [unwired: 11 in]
              }
            }
            n29 = call "set_report_class.vi"("error in (no error)"=w57, "UI_out in"=w58) -> ("error out"=w56:errorcluster, "UI_out out"=w55:T1)  [unwired: 7 in]
            n30 = call "init_instruments.vi"("error in (no error)"=w56, "UI_in"=w55) -> ("error out"=w60:errorcluster, "UI_out"=w61:T1)  [unwired: 8 in]
          }
          event "calibration": Value Change {
            n31 = event-data() -> ()  [unwired: 1 in, 6 out]
            n32 = call "init_measuring_devices.vi"("error in (no error)"=w119, "UI"=w109) -> ("error out"=w102:errorcluster, "UI out"=w101:T1)  [unwired: 8 in]
            n33 = Unbundle By Name(w101) -> ("boc_type"=w87:T3, "channel_timeout_sec"=w108:dbl)
            n34 = call "Reset cal U(SubVI).vi"("boc_type"=w87, "error in"=w102, "ResetKcoef"=TRUE, "ResetOffset"=TRUE, "paramUnicorn 2"=w118) -> ("error out"=w121:errorcluster, "Array out"=w114:sgl[][], "paramUnicorn 3"=w120:T10)  [unwired: 4 in]
            n35 = call "device_setup_tables.vi"("error in (no error)"=w121, "Enum"=w87, "paramUnicorn 3"=w120) -> ("error out"=w116:errorcluster, "paramUnicorn 2"=w117:T10)  [unwired: 7 in]
            n36 = call "device_set_timeout.vi"("error in (no error)"=w116, "Значение параметра"=w108, "paramUnicorn in"=w117) -> ("error IO"=w115:errorcluster, "ParamOut"=w112:T10)  [unwired: 7 in]
            n37 = call "boc_tablo_0_measurment.vi"("error in (no error)"=w115, "UI in"=w101, "Param_in"=w112) -> ("error out"=w96:errorcluster, "measured_value"=w77:dbl[], "UI out"=w95:T1, "Param_out"=w110:T10, "DC"=w90:dbl[], "progress"=→"Slide":u8, "RMS"=w74:dbl[], "plot"=w80:waveform(sgl)[])  [unwired: 1 in]
            "Waveform Graph - Dark" <- w80
            n38 = call "calculate_rms_coef.vi"("Array 2"=w80, "DC"=w90, "measured_value"=w77) -> ("coef_values"=w76:dbl[], "RMS values"=w75:dbl[])  [unwired: 7 in]
            n39 = call "write_calibr_result_table.vi"("new element/subarray"=w77, "error in (no error)"=w96, "Enum"=calibr_table_rows."measured", "UI in"=w95) -> ("error out"=w100:errorcluster, "UI_out"=w98:T1)  [unwired: 4 in]
            n40 = call "write_calibr_result_table.vi"("new element/subarray"=w90, "error in (no error)"=w100, "Enum"=calibr_table_rows."dc_before", "UI in"=w98) -> ("error out"=w99:errorcluster, "UI_out"=w97:T1)  [unwired: 4 in]
            n41 = call "calculate_abs.vi"("RMS"=w74, "measured_value"=w77) -> ("Array"=w83:dbl[])  [unwired: 9 in]
            n42 = call "write_calibr_result_table.vi"("new element/subarray"=w75, "error in (no error)"=w99, "Enum"=calibr_table_rows."rms_before", "UI in"=w97) -> ("error out"=w78:errorcluster, "UI_out"=w79:T1)  [unwired: 4 in]
            n43 = call "write_calibr_result_table.vi"("new element/subarray"=w83, "error in (no error)"=w78, "Enum"=calibr_table_rows."abs_before", "UI in"=w79) -> ("error out"=w82:errorcluster, "UI_out"=w81:T1)  [unwired: 4 in]
            n44 = call "write_calibr_result_table.vi"("new element/subarray"=w76, "error in (no error)"=w82, "Enum"=calibr_table_rows."rms_result", "UI in"=w81) -> ("error out"=w86:errorcluster, "UI_out"=w89:T1)  [unwired: 4 in]
            n45 = call "fil_device_cal_table.vi"("error_in"=w86, "income_table"=w114, "DC"=w90, "RMS"=w76) -> ("error_out"=w85:errorcluster, "result_table"=w103:sgl[][])  [unwired: 6 in]
            "output array" <- w103
            n46 = call "BOC_table_DC_RMS_write.vi"("Param_in"=w110, "boc_type"=w87, "table_in"=w103, "error in (no error)"=w85) -> ("param_out"=w105:T10, "error out"=w107:errorcluster)  [unwired: 4 in]
            n47 = call "save_in_flash_dialog.vi"("error in (no error)"=w107, "paramUnicorn_in"=w105) -> ("error out"=w106:errorcluster, "paramUnicorn_out"=w104:T10)  [unwired: 8 in]
            n48 = call "reset_devices.vi"("error in (no error)"=w106, "ui_input"=w89) -> ("error out"=w73:errorcluster, "UI_out"=w72:T1)  [unwired: 8 in]
          }
          event "check_calibr": Value Change {
            n49 = event-data() -> ()  [unwired: 1 in, 6 out]
            n50 = call "generator_init.vi"("error in (no error)"=w149, "UI in"=w148) -> ("error out"=w153:errorcluster, "UI out"=w154:T1)  [unwired: 8 in]
            n51 = call "voltmetr_init.vi"("error in (no error)"=w153, "UI in"=w154) -> ("error out"=w147:errorcluster, "UI out"=w143:T1)  [unwired: 8 in]
            n52 = Unbundle By Name(w143) -> ("channel_timeout_sec"=w150:dbl)
            n53 = call "device_set_timeout.vi"("error in (no error)"=w147, "Значение параметра"=w150, "paramUnicorn in"=w146) -> ("error IO"=w152:errorcluster, "ParamOut"=w151:T10)  [unwired: 7 in]
            n54 = call "boc_tablo_0_measurment.vi"("error in (no error)"=w152, "UI in"=w143, "Param_in"=w151) -> ("error out"=w134:errorcluster, "measured_value"=w133:dbl[], "UI out"=w135:T1, "Param_out"=w145:T10, "DC"=w126:dbl[], "progress"=→"Slide 2":u8, "RMS"=w125:dbl[], "plot"=→"Waveform Graph - Dark 2":waveform(sgl)[])  [unwired: 1 in]
            n55 = call "write_calibr_result_table.vi"("new element/subarray"=w133, "error in (no error)"=w134, "Enum"=calibr_table_rows."measured", "UI in"=w135) -> ("error out"=w142:errorcluster, "UI_out"=w140:T1)  [unwired: 4 in]
            n56 = call "write_calibr_result_table.vi"("new element/subarray"=w126, "error in (no error)"=w142, "Enum"=calibr_table_rows."dc_after", "UI in"=w140) -> ("error out"=w141:errorcluster, "UI_out"=w139:T1)  [unwired: 4 in]
            n57 = call "calculate_abs.vi"("RMS"=w125, "measured_value"=w133) -> ("Array"=w128:dbl[])  [unwired: 9 in]
            n58 = call "write_calibr_result_table.vi"("new element/subarray"=w125, "error in (no error)"=w141, "Enum"=calibr_table_rows."rms_after", "UI in"=w139) -> ("error out"=w132:errorcluster, "UI_out"=w131:T1)  [unwired: 4 in]
            n59 = call "write_calibr_result_table.vi"("new element/subarray"=w128, "error in (no error)"=w132, "Enum"=calibr_table_rows."abs_after", "UI in"=w131) -> ("error out"=w129:errorcluster, "UI_out"=w130:T1)  [unwired: 4 in]
            n60 = call "reset_devices.vi"("error in (no error)"=w129, "ui_input"=w130) -> ("error out"=w122:errorcluster, "UI_out"=w144:T1)  [unwired: 8 in]
          }
          event "freq_character": Value Change {
            # "Замена измеренного напряжения вольтметром\nна частоте 0.5 и 2 Гц"
            n61 = event-data() -> ()  [unwired: 1 in, 6 out]
            n62 = call "generator_init.vi"("error in (no error)"=w183, "UI in"=w185) -> ("error out"=w186:errorcluster, "UI out"=w187:T1)  [unwired: 8 in]
            n63 = call "voltmetr_init.vi"("error in (no error)"=w186, "UI in"=w187) -> ("error out"=w166:errorcluster, "UI out"=w184:T1)  [unwired: 8 in]
            n64 = call "device_set_timeout.vi"("error in (no error)"=w166, "Значение параметра"=sgl 2.0, "paramUnicorn in"=w164) -> ("error IO"=w165:errorcluster, "ParamOut"=w163:T10)  [unwired: 7 in]
            n65 = for {
              tunnel: "freq_values" -> [w192] mode=indexing
              tunnel: w184 -> [w205]
              tunnel: w165 -> [w204]
              tunnel: w163 -> [w189]
              tunnel: [w190] -> w176 mode=indexing
              tunnel: [w191] -> w174 mode=indexing
              tunnel: [w194] -> w182
              tunnel: [w195] -> w159
              tunnel: [w193] -> w177
              n66 = call "generator_set_values.vi"("error in (no error)"=w204, "Amplitude (1.0 Vpp)"=3.5, "freq_value"=w192, "UI in"=w205) -> ("error out"=w201:errorcluster, "UI_out"=w202:T1)  [unwired: 6 in]
              n67 = call "volmetr_auto_filter_freq.vi"("error in (no error)"=w201, "measure_freq_value"=w192, "UI"=w202) -> ("error out"=w188:errorcluster, "output cluster"=w200:T1)  [unwired: 7 in]
              n68 = call "boc_tablo_0_measurment.vi"("error in (no error)"=w188, "delay_before_measure"=3.0, "UI in"=w200, "Param_in"=w189) -> ("error out"=w193:errorcluster, "measured_value"=w196:dbl[], "UI out"=w195:T1, "Param_out"=w194:T10, "RMS"=w190:dbl[])  [unwired: 3 out]
              n69 = Less?(x=w192, y=3.0) -> (x < y?=w197:bool)
              n70 = case shown="True" w197 {
                tunnel: [w206 w209] -> w191
                tunnel: w196 -> [w206 w210]
                frame False {
                }
                frame True {
                  n71 = Array Size(array=w210) -> (size(s)=w208:i32)
                  n72 = Initialize Array(3.5 ("element"), w208) -> (w209:dbl[])
                }
              }
            }
            n73 = Index Array(array=w174, index (row)=2) -> (element=w169:dbl[])  [unwired: 1 in]
            n74 = Unbundle By Name(w159) -> ("Report.lvclass"=w161:refnum<class "Report.lvclass">)
            n75 = Replace Array Subset(array=w174, new element=w169, index (row)=0) -> (w170:dbl[][])  [unwired: 1 in]
            n76 = Replace Array Subset(array=w170, new element=w169, index (row)=1) -> (w168:dbl[][])  [unwired: 1 in]
            n77 = call "check_result.vi"("RMS"=w176, "measured_value"=w168, "tolerance_list"="tolerance_list") -> ("Array"=→"Array 2":bool[][])  [unwired: 8 in]
            n78 = call "assembly_result_table_freq_char.vi"("error_in"=w177, "freq_values"="freq_values", "measured_value"=w168, "RMS"=w176) -> ("error_out"=w158:errorcluster, "result_table_voltage"=w162:dbl[][])  [unwired: 6 in]
            "result_table_freq" <- w162
            n79 = Number To Fractional String(number=w162) -> (F-format string=w160:string[][])  [unwired: 3 in]
            n80 = call-dynamic "Write freq_char_table.vi"("error in (no error)"=w158, "freq_char_table"=w160, "Report in"=w161) -> ("error out"=w157:errorcluster, "Report out"=w156:refnum<class "Report.lvclass">)  [unwired: 7 in]
            n81 = Bundle By Name(cluster=w159, "Report.lvclass"=w156) -> (w155:T1)
            n82 = call "reset_devices.vi"("error in (no error)"=w157, "ui_input"=w155) -> ("error out"=w178:errorcluster, "UI_out"=w181:T1)  [unwired: 8 in]
          }
          event "volt_meas": Value Change {
            w211 = u16 1 items=["50 Ohms", "High Impedance"] ("Impedance (0: 50 Ohms)")
            n83 = event-data() -> ()  [unwired: 1 in, 6 out]
            n84 = call "generator_init.vi"("error in (no error)"=w220, "Impedance (0: 50 Ohms)"=w211, "UI in"=w221) -> ("error out"=w237:errorcluster, "UI out"=w236:T1)  [unwired: 7 in]
            n85 = call "voltmetr_init.vi"("error in (no error)"=w237, "UI in"=w236) -> ("error out"=w226:errorcluster, "UI out"=w223:T1)  [unwired: 8 in]
            n86 = call "device_set_timeout.vi"("error in (no error)"=w226, "Значение параметра"=sgl 2.0, "paramUnicorn in"=w225) -> ("error IO"=w222:errorcluster, "ParamOut"=w224:T10)  [unwired: 7 in]
            n87 = for {
              tunnel: "volt_values" -> [w243] mode=indexing
              tunnel: w223 -> [w247]
              tunnel: w222 -> [w246]
              tunnel: w224 -> [w248]
              tunnel: [w252] -> w231 mode=indexing
              tunnel: [w251] -> w230 mode=indexing
              tunnel: [w254] -> w235
              tunnel: [w255] -> w217
              tunnel: [w253] -> w232
              n88 = call "calculate_trnsformator_coef.vi"("error in (no error)"=w246, "voltage"=w243, "UI in"=w247) -> ("error out"=w245:errorcluster, "koef"=w240:dbl, "UI out 2"=w241:T1)  [unwired: 6 in]
              n89 = Divide(x=w243, y=w240) -> (x/y=w242:dbl)
              n90 = call "generator_set_values.vi"("error in (no error)"=w245, "Amplitude (1.0 Vpp)"=w242, "freq_value"=160.0, "UI in"=w241) -> ("error out"=w257:errorcluster, "UI_out"=w258:T1)  [unwired: 6 in]
              n91 = call "volmetr_auto_filter_freq.vi"("error in (no error)"=w257, "measure_freq_value"=160.0, "UI"=w258) -> ("error out"=w249:errorcluster, "output cluster"=w256:T1)  [unwired: 7 in]
              n92 = call "boc_tablo_0_measurment.vi"("error in (no error)"=w249, "delay_before_measure"=3.0, "UI in"=w256, "Param_in"=w248) -> ("error out"=w253:errorcluster, "measured_value"=w251:dbl[], "UI out"=w255:T1, "Param_out"=w254:T10, "RMS"=w252:dbl[])  [unwired: 3 out]
            }
            n93 = call "assembly_result_table_volt_char.vi"("error_in"=w232, "measured_value"=w230, "RMS"=w231) -> ("error_out"=w215:errorcluster, "result_table_voltage"=w229:dbl[][])  [unwired: 7 in]
            n94 = Unbundle By Name(w217) -> ("Report.lvclass"=w218:refnum<class "Report.lvclass">)
            n95 = Number To Fractional String(number=w229, precision (6)=i16 4) -> (F-format string=w219:string[][])  [unwired: 2 in]
            "F-format string 2" <- w219
            n96 = call "check_result.vi"("RMS"=w231, "measured_value"=w230, "tolerance_list"="tolerance_list 2") -> ("Array"=→"check_volt_result":bool[][])  [unwired: 8 in]
            n97 = call-dynamic "Write range_AC_check.vi"("error in (no error)"=w215, "range_AC_check"=w219, "Report in"=w218) -> ("error out"=w212:errorcluster, "Report out"=w213:refnum<class "Report.lvclass">)  [unwired: 7 in]
            n98 = Bundle By Name(cluster=w217, "Report.lvclass"=w213) -> (w216:T1)
            n99 = call "reset_devices.vi"("error in (no error)"=w212, "ui_input"=w216) -> ("error out"=w234:errorcluster, "UI_out"=w214:T1)  [unwired: 8 in]
          }
          event "meas_low_voltage_ac_char": Value Change {
            n100 = event-data() -> ()  [unwired: 1 in, 6 out]
            n101 = call "generator_init.vi"("error in (no error)"=w262, "UI in"=w261) -> ("error out"=w285:errorcluster, "UI out"=w284:T1)  [unwired: 8 in]
            n102 = call "voltmetr_init.vi"("error in (no error)"=w285, "UI in"=w284) -> ("error out"=w276:errorcluster, "UI out"=w274:T1)  [unwired: 8 in]
            n103 = call "device_set_timeout.vi"("error in (no error)"=w276, "Значение параметра"=sgl 2.0, "paramUnicorn in"=w260) -> ("error IO"=w273:errorcluster, "ParamOut"=w275:T10)  [unwired: 7 in]
            n104 = for {
              tunnel: "volt_values 2" -> [w290] mode=indexing
              tunnel: w274 -> [w289]
              tunnel: w273 -> [w288]
              tunnel: w275 -> [w292]
              tunnel: [w296] -> w281 mode=indexing
              tunnel: [w295] -> w280 mode=indexing
              tunnel: [w298] -> w263
              tunnel: [w299] -> w272
              tunnel: [w297] -> w282
              n105 = call "generator_set_values.vi"("error in (no error)"=w288, "Amplitude (1.0 Vpp)"=w290, "freq_value"=160.0, "UI in"=w289) -> ("error out"=w301:errorcluster, "UI_out"=w302:T1)  [unwired: 6 in]
              n106 = call "volmetr_auto_filter_freq.vi"("error in (no error)"=w301, "measure_freq_value"=160.0, "UI"=w302) -> ("error out"=w293:errorcluster, "output cluster"=w300:T1)  [unwired: 7 in]
              n107 = call "boc_tablo_0_measurment.vi"("error in (no error)"=w293, "delay_before_measure"=3.0, "UI in"=w300, "Param_in"=w292) -> ("error out"=w297:errorcluster, "measured_value"=w295:dbl[], "UI out"=w299:T1, "Param_out"=w298:T10, "RMS"=w296:dbl[])  [unwired: 3 out]
            }
            n108 = call "assembly_result_table_volt_char.vi"("error_in"=w282, "measured_value"=w280, "RMS"=w281) -> ("error_out"=w267:errorcluster, "result_table_voltage"=w279:dbl[][])  [unwired: 7 in]
            n109 = Unbundle By Name(w272) -> ("Report.lvclass"=w269:refnum<class "Report.lvclass">)
            n110 = Number To Fractional String(number=w279, precision (6)=i16 6) -> (F-format string=w268:string[][])  [unwired: 2 in]
            "F-format string" <- w268
            n111 = call "check_result.vi"("RMS"=w281, "measured_value"=w280, "tolerance_list"="tolerance_list 4") -> ("Array"=→"check_volt_result 2":bool[][])  [unwired: 8 in]
            n112 = call-dynamic "Write range_AC_check_low_voltage.vi"("error in (no error)"=w267, "range_AC_check_low_voltage"=w268, "Report in"=w269) -> ("error out"=w266:errorcluster, "Report out"=w270:refnum<class "Report.lvclass">)  [unwired: 7 in]
            n113 = Bundle By Name(cluster=w272, "Report.lvclass"=w270) -> (w271:T1)
            n114 = call "reset_devices.vi"("error in (no error)"=w266, "ui_input"=w271) -> ("error out"=w265:errorcluster, "UI_out"=w264:T1)  [unwired: 8 in]
          }
          event "curent_calibr": Value Change {
            n115 = event-data() -> ()  [unwired: 1 in, 6 out]
            n116 = call "voltmetr_init.vi"("UI in"=w342) -> ("error out"=w313:errorcluster, "UI out"=w314:T1)  [unwired: 9 in]
            n117 = call "voltmetr_setup_current_dc.vi"("error in (no error)"=w313, "UI in"=w314) -> ("error out"=w311:errorcluster, "UI out"=w312:T1)  [unwired: 8 in]
            n118 = call "reset_I_settings.vi"("error in"=w311, "paramUnicorn_in"=w355) -> ("error out"=w354:errorcluster, "table_length"=w328:i32, "result_table"=w352:sgl[][], "paramUnicorn_out"=w353:T10)  [unwired: 6 in]
            n119 = call "set_test_mod.vi"("paramUnicorn_in"=w353, "UI"=w312, "table_length"=w328, "error in (no error)"=w354) -> ("paramUnicorn_out"=w339:T10, "UI_out"=w338:T1, "error out"=w337:errorcluster)  [unwired: 4 in]
            n120 = call "set_I_and_measure.vi"("table_length"=w328, "ISetOffset_mA"=sgl 4.0, "error in (no error)"=w337, "UI in"=w338, "paramUnicorn_in"=w339) -> ("error out"=w332:errorcluster, "result"=w331:dbl[], "UI out"=w333:T1, "paramUnicorn_out out"=w334:T10)  [unwired: 3 in]
            "first_meas" <- w331
            n121 = call "set_I_and_measure.vi"("table_length"=w328, "ISetOffset_mA"=sgl 20.0, "error in (no error)"=w332, "UI in"=w333, "paramUnicorn_in"=w334) -> ("error out"=w350:errorcluster, "result"=w330:dbl[], "UI out"=w321:T1, "paramUnicorn_out out"=w322:T10)  [unwired: 3 in]
            "second_meas" <- w330
            n122 = call "calculate_I_offset.vi"("error_in"=w350, "second_meas"=w330, "first_meas"=w331, "result_table in"=w352) -> ("error_out"=w349:errorcluster, "result_table out"=w348:sgl[][])  [unwired: 6 in]
            n123 = call "0x53_Write_table_data.vi"("error in"=w349, "Номер табличного параметра 2"=9, "ArrayIn"=w348, "paramUnicorn"=w322) -> ("error out"=w326:errorcluster, "paramUnicorn 2"=w327:T10)  [unwired: 4 in, 2 out]
            n124 = call "set_I_and_measure.vi"("table_length"=w328, "ISetOffset_mA"=sgl 15.0, "error in (no error)"=w326, "UI in"=w321, "paramUnicorn_in"=w327) -> ("error out"=w325:errorcluster, "result"=w324:dbl[], "UI out"=w320:T1, "paramUnicorn_out out"=w323:T10)  [unwired: 3 in]
            n125 = call "calc_I_coef.vi"("error_in"=w325, "result_table in"=w348, "meased_values"=w324) -> ("error_out"=w347:errorcluster, "result_calibration_table"=w341:sgl[][])  [unwired: 7 in]
            "result_calibration_table" <- w341
            n126 = call "0x53_Write_table_data.vi"("error in"=w347, "Номер табличного параметра 2"=9, "ArrayIn"=w341, "paramUnicorn"=w323) -> ("error out"=w344:errorcluster, "paramUnicorn 2"=w345:T10)  [unwired: 4 in, 2 out]
            n127 = for {
              tunnel: "I_control_values" -> [w356] mode=indexing
              tunnel: w345 -> [w364]
              tunnel: w344 -> [w360]
              tunnel: [w357] -> w310 mode=indexing
              tunnel: [w359] -> w307
              tunnel: [w358] -> w343
              tunnel: [w361] -> w317
              tunnel: w328 -> [w362]
              tunnel: w320 -> [w363]
              n128 = call "set_I_and_measure.vi"("table_length"=w362, "ISetOffset_mA"=w356, "error in (no error)"=w360, "UI in"=w363, "paramUnicorn_in"=w364) -> ("error out"=w359:errorcluster, "result"=w357:dbl[], "UI out"=w358:T1, "paramUnicorn_out out"=w361:T10)  [unwired: 3 in]
            }
            n129 = call "assembly_result_table_I_cal.vi"("error_in"=w307, "result"=w310, "I_control_values"="I_control_values") -> ("error_out"=w306:errorcluster, "result_table"=→"result_table":dbl[][])  [unwired: 7 in]
            n130 = call "check_result_I_calibr.vi"("error_in"=w306, "I_control_values"="I_control_values", "tolerance_list_I_correction"="tolerance_list_I_correction", "result"=w310) -> ("error_out"=w318:errorcluster, "Array 2"=→"check_result":bool[][])  [unwired: 6 in]
            n131 = call "reset_devices.vi"("error in (no error)"=w318, "ui_input"=w343) -> ("error out"=w315:errorcluster, "UI_out"=w305:T1)  [unwired: 8 in]
            n132 = call "save_in_flash_dialog.vi"("error in (no error)"=w315, "paramUnicorn_in"=w317) -> ("error out"=w304:errorcluster, "paramUnicorn_out"=w316:T10)  [unwired: 8 in]
          }
          event "dc_voltage_measure": Value Change {
            n133 = event-data() -> ()  [unwired: 1 in, 6 out]
            n134 = Unbundle By Name(w386) -> ("voltmetr"=w388:refnum<visa-resource-name>)
            n135 = call <instrlib>:"Reset.vi"("error in (no error)"=w387, "VISA resource name"=w388) -> ("error out"=w385:errorcluster)  [unwired: 8 in, 1 out]
            n136 = call "determine_positive_channel.vi"("error in (no error)"=w385, "UI in"=w386) -> ("error out"=w384:errorcluster, "determined_channels"=w389:T19, "UI out"=w381:T1)  [unwired: 7 in]
            n137 = call "boc_reset_tuned_by_user_table.vi"("error in (no error)"=w384, "UI in"=w381, "paramUnicorn"=w383) -> ("error out"=w391:errorcluster, "UI_out"=w380:T1, "paramUnicorn out"=w382:T10)  [unwired: 5 in, 1 out]
            n138 = Initialize Array(0.0 ("element"), 12 ("dimension size"), 37 ("dimension size")) -> (w376:dbl[][])
            n139 = for {
              shift-right: [w405] -> w392
              shift-left: w382 -> [w413]
              shift-right: [w398] -> w369
              shift-left: w391 -> [w407]
              shift-right: [w404] -> w367
              shift-left: w380 -> [w411]
              tunnel: "voltage" -> [w403] mode=indexing
              tunnel: w389 -> [w408]
              shift-right: [w401] -> _
              shift-left: w376 -> [w402]
              tunnel: [w397] -> w374 mode=indexing
              tunnel: [w394] -> w373 mode=indexing
              tunnel: [w396] -> w370
              i -> [w400]
              stop <- w398 stop-if-true
              n140 = call "convert_voltage_to_motech.vi"("error_in"=w407, "determined_channels"=w408, "voltage"=w403) -> ("error_out"=w406:errorcluster, "motech_set_value"=w409:T7)  [unwired: 7 in]
              n141 = call "set_dc_voltage.vi"("error in (no error)"=w406, "motech_set_value"=w409, "UI in"=w411) -> ("error out"=w410:errorcluster, "UI out 2"=w412:T1)  [unwired: 7 in]
              n142 = call "measure_volt_dc.vi"("error in (no error)"=w410, "UI out 3"=w412, "paramUnicorn in"=w413) -> ("error out"=w399:errorcluster, "measured"=w395:dbl[], "UI out 2"=w404:T1, "paramUnicorn 2"=w405:T10, "boc_data"=w397:sgl[])  [unwired: 4 in]
              n143 = Absolute Value(x=w395) -> (abs(x)=w394:dbl[])
              n144 = call "compile_table.vi"("income_array"=w402, "row_number"=w400, "error_in"=w399, "value"=w403, "boc-data"=w397, "measured"=w395) -> ("error_out"=w398:errorcluster, "table"=w396:string[][], "output_data"=w401:dbl[][])  [unwired: 3 in]
              "Table Control" <- w396
            }
            n145 = Unbundle By Name(w367) -> ("Report.lvclass"=w371:refnum<class "Report.lvclass">)
            n146 = call-dynamic "Write range_DC_check.vi"("error in (no error)"=w369, "range_DC_check"=w370, "Report in"=w371) -> ("error out"=w368:errorcluster, "Report out"=w365:refnum<class "Report.lvclass">)  [unwired: 7 in]
            n147 = call "check_result.vi"("RMS"=w374, "measured_value"=w373, "tolerance_list"="tolerance_list 3") -> ("Array"=→"Array 3":bool[][])  [unwired: 8 in]
            n148 = Bundle By Name(cluster=w367, "Report.lvclass"=w365) -> (w366:T1)
          }
          event "set_V": Value Change {
            n149 = event-data() -> ()  [unwired: 1 in, 6 out]
            n150 = Unbundle By Name(w419) -> ("DC_power_supply.lvclass"=w421:refnum<class "DC_power_supply.lvclass">)
            n151 = call-dynamic "set_channel_params.vi"("error in (no error)"=w416, "motech_set_value"="motech_set_value", "DC_power_supply in"=w421) -> ("error out"=w415:errorcluster, "DC_power_supply out"=w420:refnum<class "DC_power_supply.lvclass">)  [unwired: 7 in]
            n152 = Bundle By Name(cluster=w419, "DC_power_supply.lvclass"=w420) -> (w418:T1)
          }
          event "avarage_Ac_input": Value Change {
            n153 = event-data() -> ()  [unwired: 1 in, 6 out]
            n154 = Unbundle By Name(w422) -> ("voltmetr"=w438:refnum<visa-resource-name>)
            n155 = call <instrlib>:"Reset.vi"("error in (no error)"=w427, "VISA resource name"=w438) -> ("error out"=w437:errorcluster)  [unwired: 8 in, 1 out]
            n156 = call "determine_positive_channel.vi"("error in (no error)"=w437, "UI in"=w422) -> ("error out"=w436:errorcluster, "determined_channels"=w439:T19, "UI out"=w434:T1)  [unwired: 7 in]
            n157 = call "boc_reset_tuned_by_user_table.vi"("error in (no error)"=w436, "UI in"=w434, "paramUnicorn"=w428) -> ("error out"=w441:errorcluster, "UI_out"=w433:T1, "paramUnicorn out"=w435:T10)  [unwired: 5 in, 1 out]
            n158 = Initialize Array(0.0 ("element"), 12 ("dimension size"), 37 ("dimension size")) -> (w429:dbl[][])
            n159 = for {
              shift-right: [w446] -> w423
              shift-left: w435 -> [w447]
              shift-right: [w450] -> w426
              shift-left: w441 -> [w457]
              shift-right: [w445] -> w425
              shift-left: w433 -> [w460]
              tunnel: "voltage 2" -> [w455] mode=indexing
              tunnel: w439 -> [w458]
              shift-right: [w452] -> _
              shift-left: w429 -> [w454]
              i -> [w451]
              stop <- w450 stop-if-true
              n160 = call "convert_voltage_to_motech.vi"("error_in"=w457, "determined_channels"=w458, "voltage"=w455) -> ("error_out"=w456:errorcluster, "motech_set_value"=w459:T7)  [unwired: 7 in]
              n161 = call "set_dc_voltage.vi"("error in (no error)"=w456, "motech_set_value"=w459, "UI in"=w460) -> ("error out"=w449:errorcluster, "UI out 2"=w448:T1)  [unwired: 7 in]
              n162 = call "check_average_AC_input.vi"("error in (no error)"=w449, "UI out 3"=w448, "paramUnicorn in"=w447) -> ("error out"=w444:errorcluster, "measured"=w442:dbl[], "UI out 2"=w445:T1, "paramUnicorn 2"=w446:T10, "boc_data"=w443:sgl[])  [unwired: 4 in]
              n163 = call "compile_table.vi"("income_array"=w454, "row_number"=w451, "error_in"=w444, "value"=w455, "boc-data"=w443, "measured"=w442) -> ("error_out"=w450:errorcluster, "table"=→"Table Control 2":string[][], "output_data"=w452:dbl[][])  [unwired: 3 in]
            }
          }
          event "check_dc_icp": Value Change {
            n164 = event-data() -> ()  [unwired: 1 in, 6 out]
            n165 = Unbundle By Name(w471) -> ("voltmetr"=w486:refnum<visa-resource-name>)
            n166 = call <instrlib>:"Reset.vi"("error in (no error)"=w484, "VISA resource name"=w486) -> ("error out"=w483:errorcluster)  [unwired: 8 in, 1 out]
            n167 = call "boc_reset_tuned_by_user_table.vi"("error in (no error)"=w483, "UI in"=w471, "paramUnicorn"=w485) -> ("error out"=w480:errorcluster, "cleaned_params"=w479:sgl[][], "UI_out"=w482:T1, "paramUnicorn out"=w470:T10)  [unwired: 5 in]
            n168 = call "boc_measure_all_channels.vi"("Function"=Function."VOLTage:DC", "error in (no error)"=w480, "paramUnicorn in"=w470, "input cluster"=w482) -> ("error out"=w477:errorcluster, "boc_values"=w463:sgl[], "paramUnicorn out"=w469:T10, "output cluster"=w478:T1, "results"=w465:dbl[])  [unwired: 3 in]
            n169 = call "meas_eidi.vi"("error in"=w477, "user_params_table"=w479, "input cluster"=w478, "paramUnicorn"=w469) -> ("error out"=w474:errorcluster, "results"=w468:dbl[][], "output cluster"=w475:T1, "paramUnicorn 2"=w476:T10, "boc_values"=w464:sgl[][])  [unwired: 3 in]
            n170 = Insert Into Array(array=w464, index (row)=0, new element=w463) -> (→"boc_values":sgl[][])  [unwired: 1 in]
            n171 = Insert Into Array(array=w468, index (row)=0, new element=w465) -> (→"output array 2":dbl[][])  [unwired: 1 in]
            n172 = call "reset_devices.vi"("error in (no error)"=w474, "ui_input"=w475) -> ("error out"=w472:errorcluster, "UI_out"=w473:T1)  [unwired: 8 in]
          }
          event "template": Value Change {
            n173 = event-data() -> ("NewVal"=w494:path)  [unwired: 1 in, 5 out]
            n174 = Unbundle By Name(w492) -> ("Report.lvclass"=w495:refnum<class "Report.lvclass">)
            n175 = call-dynamic "set_template_file.vi"("error in (no error)"=w493, "Path"=w494, "Report in"=w495) -> ("error out"=w489:errorcluster, "Report out"=w491:refnum<class "Report.lvclass">)  [unwired: 7 in]
            n176 = Bundle By Name(cluster=w492, "Report.lvclass"=w491) -> (w490:T1)
          }
          event "report": Value Change {
            n177 = event-data() -> ("NewVal"=w503:path)  [unwired: 1 in, 5 out]
            n178 = Unbundle By Name(w501) -> ("Report.lvclass"=w504:refnum<class "Report.lvclass">)
            n179 = call "Write output_file_path.vi"("error in (no error)"=w502, "output_file_path"=w503, "Report in"=w504) -> ("error out"=w499:errorcluster, "Report out"=w500:refnum<class "Report.lvclass">)  [unwired: 7 in]
            n180 = Bundle By Name(cluster=w501, "Report.lvclass"=w500) -> (w498:T1)
          }
          event "export_report": Value Change {
            n181 = event-data() -> ()  [unwired: 1 in, 6 out]
            n182 = Unbundle By Name(w513) -> ("Report.lvclass"=w517:refnum<class "Report.lvclass">)
            n183 = call-dynamic "add_amp_char_to_report.vi"("error in (no error)"=w511, "Report in"=w517) -> ("error out"=w510:errorcluster, "Report out"=w516:refnum<class "Report.lvclass">)  [unwired: 8 in]
            n184 = call-dynamic "add_freq_char_to_report.vi"("error in (no error)"=w510, "Report in"=w516) -> ("error out"=w509:errorcluster, "Report out"=w515:refnum<class "Report.lvclass">)  [unwired: 8 in]
            n185 = call-dynamic "add_range_AC_check_to_report.vi"("error in (no error)"=w509, "Report in"=w515) -> ("error out"=w508:errorcluster, "Report out"=w514:refnum<class "Report.lvclass">)  [unwired: 8 in]
            n186 = call-dynamic "add_range_DC_check_to_report.vi"("error in (no error)"=w508, "Report in"=w514) -> ("error out"=w507:errorcluster, "Report out"=w512:refnum<class "Report.lvclass">)  [unwired: 8 in]
            n187 = Bundle By Name(cluster=w513, "Report.lvclass"=w512) -> (w506:T1)
          }
          event Timeout {
            n188 = event-data() -> ()  [unwired: 1 in, 3 out]
            n189 = Unbundle By Name(w520) -> ("conParam.TCP_conn"=→"Con":bool)
          }
          event "generator": Value Change {
            n190 = event-data() -> ("NewVal"=w529:refnum<visa-resource-name>)  [unwired: 1 in, 5 out]
            n191 = call <instrlib>:"Initialize.vi"("error in (no error)"=w528, "VISA resource name"=w529) -> ("error out"=w524:errorcluster, "VISA resource name out"=w526:refnum<visa-resource-name>)  [unwired: 8 in]
            n192 = Bundle By Name(cluster=w527, "generator"=w526) -> (w525:T1)
          }
          event "dc_power_supply": Value Change {
            n193 = event-data() -> ("NewVal"=w532:refnum<visa-resource-name>)  [unwired: 1 in, 5 out]
            n194 = Unbundle By Name(w537) -> ("DC_power_supply.lvclass"=w534:refnum<class "DC_power_supply.lvclass">)
            n195 = call-dynamic "set_port.vi"("error in (no error)"=w533, "VISA resource name"=w532, "DC_power_supply in"=w534) -> ("error out"=w531:errorcluster, "DC_power_supply out"=w530:refnum<class "DC_power_supply.lvclass">)  [unwired: 7 in]
            n196 = Bundle By Name(cluster=w537, "DC_power_supply.lvclass"=w530) -> (w536:T1)
          }
          event "voltmetr": Value Change {
            n197 = event-data() -> ("NewVal"=w543:refnum<visa-resource-name>)  [unwired: 1 in, 5 out]
            n198 = call <instrlib>:"Initialize.vi"("error in (no error)"=w541, "VISA resource name"=w543) -> ("error out"=w540:errorcluster, "VISA resource name out"=w542:refnum<visa-resource-name>)  [unwired: 7 in, 1 out]
            n199 = Bundle By Name(cluster=w544, "voltmetr"=w542) -> (w539:T1)
          }
        }
        n200 = call "error_handler.vi"("error in (no error)"=w39) -> ("error out"=w40:errorcluster)  [unwired: 10 in]
      }
    }
  }
  "error out" <- w3
  n201 = local write "Array"(dbl[][] [] ("Array")) -> ()
